vi "VP_RT_ModTrans.vi"() -> ()   [LabVIEW 2015]
uses:
  Local or Remote.ctl
  State Enum.ctl
  Command Enum.ctl
  Controller Type.ctl
  EPICS Command Control.ctl
  Plot options enum.ctl
  Stream SM states.ctl
  <vilib>/Platform/TimedLoop/XDataNode/timing_clust.ctl
  <vilib>/Platform/TimedLoop/XDataNode/nitl_modes.ctl
  <vilib>/Platform/TimedLoop/XDataNode/wakeup.ctl
  Data Write Control.ctl
  Data stream writer.vi
  <vilib>/Utility/error.llb/Error Cluster From Error Code.vi
  <vilib>/rvi/errors/niLvFpgaAdjustHostInterfaceError.vi
  <vilib>/rvi/interface/common/niFpgaWaitOnOcc.vi
  <vilib>/FPGAPlugInAG/Dynamic/niLvFpga_Reset_Dynamic.vi
  <vilib>/FPGAPlugInAG/Dynamic/niLvFpga_Abort_Dynamic.vi
  <vilib>/FPGAPlugInAG/Dynamic/niLvFpga_Close_Dynamic.vi
  Error stream writer.vi
  <vilib>/Platform/TimedLoop/XDataNode/XDataNode.xnode
  <vilib>/rvi/interface/nirviReadWriteControl/nirviReadWriteControl.xnode
  <vilib>/rvi/interface/nirviMethod/nirviMethod.xnode
  <vilib>/rvi/interface/nirviCloseFPGA/nirviCloseFPGA.xnode
  <vilib>/Platform/TimedLoop/XDataNode/XDNodeRunTimeDep.lvlib
  <vilib>/rvi/errors/niLvFpgaMergeErrorWithErrorCode.vi
  NiFpgaLv.dll
  <vilib>/rvi/interface/Simulation/niFpgaSimulationCallBeginRW.vi
  <vilib>/rvi/Analysis/host/Public/NI_FpgaMspHost.lvlib
  <vilib>/FPGAPlugInAG/Dynamic/niLvFpga_StopFifo_Dynamic.vi
  <vilib>/FPGAPlugInAG/Dynamic/niLvFpga_ReadFifo_Dynamic.vi
  <vilib>/NI_Real-Time Target Support.lvlib
  <vilib>/FPGAPlugInAG/Dynamic/niLvFpga_ConfigureFifo_Dynamic.vi
  <vilib>/FPGAPlugInAG/Dynamic/niLvFpga_StartFifo_Dynamic.vi
  <resource>/objmgr/ni.dex.rc
panel:
  in  "Tab Control":T1(tab)
  in  "Controller Type":T2
  in  "X Ramp Start (nm)":fxp<+/-,32,16>
  in  "X Ramp End (nm)":fxp<+/-,32,16>=500.0
  in  "Y Ramp Start (nm)":fxp<+/-,32,16>
  in  "Y Ramp End (nm)":fxp<+/-,32,16>=-500.0
  in  "Y Step Size (nm)":fxp<+/-,32,16>=50.0
  in  "X Step Size (nm)":fxp<+/-,32,16>=50.0
  in  "System Loop Type":enum16{"Open Loop", "Closed Loop"}(ring)=enum."Closed Loop"
  in  "DT Frequency (Hz)":dbl=3000.0 format="%#_6p"
  in  "DT duty cycle (%)":dbl=88.0 min=0.0 max=100.0 step=1.0
  in  "Max radius":fxp<+/-,32,16>=500.0
  in  "Spiral Step Size":fxp<+/-,32,16>=50.0
  in  "Scan Geometry":T3(ring)
  in  "Inner Scan axis":enum16{"X", "Y"}(ring)
  in  "Rotation Direction":enum16{"Clockwise", "Anti-clockwise"}(ring)
  in  "Radial direction":enum16{"Outward", "Inward"}(ring)
  out "Trajectory Completed":bool
  out "XY Ref":cluster{dbl[], dbl[]}[](graph)
  out "Elements Available in FIFO":u32(graph)
  out "Elements Remaining in FIFO":u32(graph)
  out "Reference and Actual positions":cluster{"t0":dbl, dbl, dbl[][]}(graph)
  in  "Timeout FPGA FIFO1":i32=40000000
  out "FIFO Timed Out":bool
  out "Stop Run":bool
  in  "Datalog Cases":T4(ring)=enum."Data Log 16"
  out "FIFO Timed Out?":bool
  out "Data Read Rate (Hz)":dbl=25000.000000000004
  out "Elements Remaining":u32
  in  "FIFO Timeout (ms)":i32=2500
  out "Actual Depth":u32=131068416
  in  "Requested Depth":u32=131068000
  in  "Fly scan loop dt":i64=250
  in  "Start Scan Loop dt":i64=50
  out "Queue is empty":bool=TRUE
  out "2iddVELO:VP:X_End_nm":dbl=2000.0
  out "2iddVELO:VP:X_Start_nm":dbl=-2000.0
  out "EPICS Execute Command":bool
  out "2iddVELO:VP:Y_Start_nm":dbl=2000.0
  out "2iddVELO:VP:Y_End_nm":dbl=-2000.0
  out "2iddVELO:VP:Y_Step_Size_nm":dbl=50.0
  out "2iddVELO:VP:X_Step_Size_nm":dbl=50.0
  out "2iddVELO:VP:Trigger_Freq_Hz":dbl=1000.0
  out "2iddVELO:VP:Trig_DutyCycle_Per":dbl=99.0
  out "Remote Mode":bool
  out "EPICS Controller Type":T2
  out "EPICS cRIO Command":T5
  out "EPICS Scan Trajectory":T3(ring)
  out "2iddVELO:VP:Max_Radius":dbl
  out "2iddVELO:VP:Spiral_Step":dbl
  out "Iteration Duration RT Timed-Loop":i64=128
  in  "Controller Time Period (uSec)":u32=40
  in  "Controller Output Time Period (uSec)":u32=40
  in  "XY Reference Time Period (uSec)":u32=40
  in  "Plant Output Time Period (uSec)":u32=40
  in  "Datalog Time Period (uSec)":u32=40
  in  "Trigger Generation Time Period (uSec)":u32=40
  in  "Z Reference Time Period (uSec)":u32=40
  in  "Stop System (Careful!!)":bool
  in  "Reset All":bool
  in  "Base name":string="base_name"
  out "Mod6/DIO3":bool
  out "Mod5/DIO3":bool
  out "Mod4/DIO3":bool
  in  "Sample Z Stage Resolution (nm)":fxp<+,33,3>=0.5
  in  "Sample Y Stage Resolution (nm)":fxp<+,33,3>=0.5
  in  "Sample X Stage Resolution (nm)":fxp<+,33,3>=0.5
  in  "Optics Z Stage Resolution (nm)":fxp<+,33,3>=0.5
  in  "Optics Y Stage Resolution (nm)":fxp<+,33,3>=0.5
  in  "Optics X Stage Resolution (nm)":fxp<+,33,3>=0.5
  in  "Sample Z Reset":bool
  in  "Sample Y Reset":bool
  in  "Sample X Reset":bool
  out "Mod6/DIO2":bool
  out "Mod6/DIO1":bool
  out "Mod6/DIO0":bool=TRUE
  out "Mod5/DIO2":bool
  out "Mod5/DIO1":bool=TRUE
  out "Mod5/DIO0":bool
  out "Mod4/DIO2":bool=TRUE
  out "Mod4/DIO1":bool
  out "Mod4/DIO0":bool=TRUE
  in  "Optics Z Reset":bool
  in  "Optics Y Reset":bool
  in  "Optics X Reset":bool
  out "Heartbeat":bool=TRUE
  in  "System command":T6
  in  "Execute":bool
  out "Last Command Executed":T6
  in  "Optics and or Sample Stage":T7(ring)
  in  "Local_Lock":bool
  out "Local or EPICS":T8
  out "Output filename":string
  out "Output path":path
  in  "cRIO data dir":string="/home/lvuser/natinst/data"
  out "RT Main Loop State":T9
  out "cRIO path":path
  out "Iteration Duration":i64
  out "EPICS rotation direction":enum16{"Clockwise", "Anti-clockwise"}(ring)
  out "EPICS radial direction":enum16{"Outward", "Inward"}(ring)
  out "EPICS Inner axis":enum16{"X", "Y"}(ring)
  out "Optics Z Stage Displacement (nm)":fxp<+/-,32,16>
  out "Optics Y Stage Displacement (nm)":fxp<+/-,32,16>
  out "Optics X Stage Displacement (nm)":fxp<+/-,32,16>=-1.0
  in  "Scan type":enum16{"Fly", "Step"}(ring)
  out "EPICS Scan Type":enum16{"Fly", "Step"}(ring)
  out "Scan Type and Geometry":T10(ring)
  out "Position Number":u32
  in  "Plot option":T11
  out "EPICS data save trigger":enum16{"Detector", "Trajectory"}(ring)
  out "Outer Loop iterations":i32
  out "Counter Loop iterations":i32
  out "Plant output loop iterations":i32
  out "Module output loop iterations":i32
  out "Trigger Generation Loop iterations":i32
  out "FIFO loop iterations":i32
  out "XY Reference Loop iterations":i32
  out "Z Reference Loop iterations":i32
  out "Controller loop iterations":i32
  out "FPGA state":T12(ring)
  out "EPICS system loop type":enum16{"Open Loop", "Closed Loop"}(ring)
  out "2iddVELO:LabView:ZPZ_Command":dbl
  out "2iddVELO:LabView:ZPY_Command":dbl
  out "2iddVELO:LabView:ZPX_Command":dbl
  out "Data sream sends":i32
  out "Error stream sends":i32
  out "Data stream writer connection":bool
  out "Error stream writer connection":bool
  out "Data stream state":T13
  out "Error stream state":T13
  in  "Data phase offset (deg)":dbl
  in  "Data frequency (Hz)":dbl=2500.0
  in  "Data duty cycle (%)":dbl=50.0
  in  "Data Trigger Reset":bool
  out "Data Frequency":fxp<+,32,0>
  out "Data Duty Cycle (periods)":fxp<+,32,0>
  out "Data Phase Offset (periods)":fxp<+,32,0>
  out "2iddVELO:VP:Data_Freq_Hz":dbl
  in  "Z-Stage Scaling Direction":fxp<+/-,3,3>=-1.0
  in  "Y-Stage Scaling Direction":fxp<+/-,3,3>=-1.0
  in  "Z-Stage nm to V Scaling":fxp<+/-,32,12>=0.0005397796630859375
  in  "Y-Stage nm to V Scaling":fxp<+/-,32,12>=0.0014200210571289062
  in  "X-Stage Scaling Direction":fxp<+/-,3,3>=-1.0
  in  "X-Stage nm to V Scaling":fxp<+/-,32,12>=0.0005359649658203125
  in  "Controller Output Lower Limit":fxp<+/-,20,5>=-5.0
  in  "Controller Output Upper Limit":fxp<+/-,20,5>=5.0
  in  "FPGA Wait Timer (ms)":u16=5
  in  "Pre-Scan pause (ms)":u32=2000
  in  "Readback Loop time between iterations (ms)":u32=10
  in  "Z Reference DC Offset (nm)":fxp<+/-,15,15>
  in  "Y Reference DC Offset (nm)":fxp<+/-,16,16>
  in  "X Reference DC Offset (nm)":fxp<+/-,16,16>
  in  "Z Reference Amplitude (nm)":fxp<+/-,40,17>
  in  "Y Reference Amplitude (nm)":fxp<+/-,40,17>=100.0
  in  "X Reference Amplitude (nm)":fxp<+/-,40,17>=100.0
  out "Trajectory frequency (periods/tick)":fxp<+,32,0>=1.25030055642128e-07 format="%#.5e"
  in  "Trajectory frequency (Hz)":dbl=25000.0 format="%#_6p"
  out "actual Traj frequency (Hz)":dbl format="%#_6p"
  in  "Data Save Flag":enum16{"Skip Data", "Save Data"}(ring)=enum."Save Data"
  in  "X Start Marker (nm)":fxp<+/-,32,16>
  in  "Y Start Marker (nm)":fxp<+/-,32,16>
  in  "Post-Scan pause (ms)":u32=2000
  in  "Detector Trigger Lower Limit (V)":fxp<+/-,20,5>
  in  "Detector Trigger Upper Limit (V)":fxp<+/-,20,5>=5.0
  out "Detector Trigger In Range?":bool=TRUE
  in  "Det Reference Amplitude (V)":fxp<+/-,40,17>=5.0
  in  "DT Reference DC Offset (V)":fxp<+/-,16,16>
  out "Det Frequency (periods/tick)":fxp<+,32,0>=7.500010542571545e-05
  out "Det Phase Offset (periods)":fxp<+,32,0>
  in  "Det Reset":bool
  out "Det Duty Cycle (periods)":fxp<+,32,0>=0.8799999998882413
  in  "Det phase offset (deg)":dbl format="%#.6g"
  out "Det Trigger Frequency (Hz)":dbl
  out "Det Trigger Duty Cycle (%)":dbl
  in  "Scaling mV to V":fxp<+,33,10>=0.001000046730041504
  out "Measured Datalog Time Period (Ticks)":u32=1600
  out "Measured Datalog Loop Rate (us)":dbl=3.9999999999999996e-05
  out "Measured Datalog Loop Rate (kHz)":dbl=25.000000000000004
  out "Measured Counter Loop Rate (us)":dbl
  out "Measured Counter Loop Rate (MHz)":dbl=inf
  out "Measured XY Reference Loop Rate (us)":dbl=3.9999999999999996e-05
  out "Measured XY Reference Loop Rate (kHz)":dbl=25.000000000000004
  out "Measured XY Reference Time Period (Ticks)":u32=1600
  out "Measured Controller Loop Rate (kHz)":dbl=25.000000000000004
  out "Measured Controller Output Loop Rate (us)":dbl=3.9999999999999996e-05
  out "Measured Controller Output Loop Rate (kHz)":dbl=25.000000000000004
  out "Measured Plant Output Loop Rate (us)":dbl=3.9999999999999996e-05
  out "Measured Plant Output Loop Rate (kHz)":dbl=25.000000000000004
  out "Measured Controller Loop Rate (us)":dbl=3.9999999999999996e-05
  out "Measured Controller Time Period (Ticks)":u32=1600
  out "Data Read Period (sec)":dbl=3.9999999999999996e-05
  out "Measured Controller Output Time Period (Ticks)":u32=1600
  out "Measured Plant Output Time Period (Ticks)":u32=1600
  out "Measured Counter Time Period (Ticks)":u32
  out "Measured Trigger Gen Time Period (Ticks)":u32=1600
  out "Measured Z Reference Time Period (Ticks)":u32=1600
  out "Measured Z Reference Loop Rate (us)":dbl=3.9999999999999996e-05
  out "Measured Z Reference Loop Rate (kHz)":dbl=25.000000000000004
  out "Number of Data Strings":i32=5
  out "Data":fxp<+/-,40,32>[](array[numeric])
  out "Measured Trigger Gen Loop Rate (us)":dbl=3.9999999999999996e-05
  out "Measured Trigger Gen Loop Rate (kHz)":dbl=25.000000000000004
  out "Z-Stage Input In Range?":bool=TRUE
  out "Y-Stage Input In Range?":bool=TRUE
  out "X-Stage Input In Range?":bool=TRUE
  out "Controller Output Upper Limit Readback":fxp<+/-,20,5>
  out "Kyy Output, Kyy*ey (V)":fxp<+/-,58,25>
  out "Controller Output Lower Limit Readback":fxp<+/-,20,5>
  out "Kxx Output, Kxx*ex (V)":fxp<+/-,58,25>
  out "Kzz Output, Kzz*ez (V)":fxp<+/-,58,25>
  in  "file path soscoeff_xx1 Hinf":path=path "/home/lvuser/natinst/controllers/Kxx_1_Gxx_matched_dow_16ord_mVpnm_cd8a3_AvTio9_X5nm_500pm_all_40us_soscof_xx1.mat"
  in  "file path sos gain SF Controller_xx1 Hinf":path=path "/home/lvuser/natinst/controllers/Kxx_1_Gxx_matched_dow_16ord_mVpnm_cd8a3_AvTio9_X5nm_500pm_all_40us_soscof_xx2.mat"
  in  "file path soscoeff_yy1 Hinf":path=path "/home/lvuser/natinst/controllers/Kyy_trial_1_Gyy_matched_dow_8ord_mVpnm_cd8a3_AvTio9_Y5nm_500pm_all_40us_soscof_yy1.mat"
  in  "file path sos gain SF Controller_yy1 Hinf":path=path "/home/lvuser/natinst/controllers/Kyy_trial_1_Gyy_matched_dow_8ord_mVpnm_cd8a3_AvTio9_Y5nm_500pm_all_40us_soscof_yy2.mat"
  in  "file path soscoeff_zz1 Hinf":path=path "/home/lvuser/natinst/controllers/Kzz_1_Gzz_matched_dow_29ord_mVpnm_cd8a3_AvTio9_Z5nm_500pm_all_40us_soscof_zz1.mat"
  in  "file path sos gain SF Controller_zz1 Hinf":path=path "/home/lvuser/natinst/controllers/Kzz_1_Gzz_matched_dow_29ord_mVpnm_cd8a3_AvTio9_Z5nm_500pm_all_40us_soscof_zz2.mat"
  in  "file path soscoeff_xx1 PID":path=path "/home/lvuser/natinst/controllers/Kxx_pid_2_Gxx_tustin_2ord_mVpnm_cd8a3_soscof_xx1.mat"
  in  "file path sos gain SF Controller_xx1 PID":path=path "/home/lvuser/natinst/controllers/Kxx_pid_2_Gxx_tustin_2ord_mVpnm_cd8a3_soscof_xx2.mat"
  in  "file path soscoeff_yy1 PID":path=path "/home/lvuser/natinst/controllers/Kyy_pid_4_Gyy_tustin_2ord_mVpnm_cd8a3_soscof_yy1.mat"
  in  "file path sos gain SF Controller_yy1 PID":path=path "/home/lvuser/natinst/controllers/Kyy_pid_4_Gyy_tustin_2ord_mVpnm_cd8a3_soscof_yy2.mat"
  in  "file path soscoeff_zz1 PID":path=path "/home/lvuser/natinst/controllers/Kzz_pid_2_Gzz_tustin_2ord_mVpnm_cd8a3_soscof_zz1.mat"
  in  "file path sos gain SF Controller_zz1 PID":path=path "/home/lvuser/natinst/controllers/Kzz_pid_2_Gzz_tustin_2ord_mVpnm_cd8a3_soscof_zz2.mat"
  out "-a01(2) xx1c":fxp<+/-,64,9>[](array[numeric])=[0.637785025840232, 0.9924182654286198, 1.8461027816316544, 0.8635404845716299, 1.0670555456779864, 1.6350703383821101, 1.6323955588345012, 1.1102241390539636, 0.0, 0.0, 0.0, 0.0, 0.0, 0.0, 0.0, 0.0, 0.0, 0.0, 0.0, 0.0]
  out "-a02(2) xx1c":fxp<+/-,64,9>[](array[numeric])=[-0.999855815746439, -0.9676991072632725, -0.9642268720534838, -0.9446498323360957, -0.9442808087139987, -0.7547983908829242, -0.6690016013017409, -0.11027986125857198, 0.0, 0.0, 0.0, 0.0, 0.0, 0.0, 0.0, 0.0, 0.0, 0.0, 0.0, 0.0]
  out "b01(2) xx1c":fxp<+/-,64,9>[](array[numeric])=[-0.6378105164532328, -1.0062332697665268, -1.8762916543815855, -0.8616288879491845, -1.0856571140792324, -1.6862585929720944, -1.743591709663851, -0.6129835805090948, 0.0, 0.0, 0.0, 0.0, 0.0, 0.0, 0.0, 0.0, 0.0, 0.0, 0.0, 0.0]
  out "b02(2) xx1c":fxp<+/-,64,9>[](array[numeric])=[0.9999102047610771, 0.9971375605901365, 0.9926840301018772, 0.9509648854364836, 0.9563369558920378, 0.7818900462139817, 0.7642575436257291, 3.0531133177191805e-16, 0.0, 0.0, 0.0, 0.0, 0.0, 0.0, 0.0, 0.0, 0.0, 0.0, 0.0, 0.0]
  out "sos gain SF Controller xx1c":fxp<+/-,42,9>=-0.1625035791657865
  out "-a01(2) yy1c":fxp<+/-,64,9>[](array[numeric])=[1.8740229377643998, 1.3096977339382483, 1.7453886241944765, 0.2668895009727739, 0.0, 0.0, 0.0, 0.0, 0.0, 0.0, 0.0, 0.0, 0.0, 0.0, 0.0, 0.0, 0.0, 0.0, 0.0, 0.0]
  out "-a02(2) yy1c":fxp<+/-,64,9>[](array[numeric])=[-0.9732703278433918, -0.5194903821190732, -0.7453924481836136, -2.7755575615628914e-17, 0.0, 0.0, 0.0, 0.0, 0.0, 0.0, 0.0, 0.0, 0.0, 0.0, 0.0, 0.0, 0.0, 0.0, 0.0, 0.0]
  out "b01(2) yy1c":fxp<+/-,64,9>[](array[numeric])=[-1.8979173162254057, -1.8463149313261074, -1.7151162246453355, -0.006444279582847878, 0.0, 0.0, 0.0, 0.0, 0.0, 0.0, 0.0, 0.0, 0.0, 0.0, 0.0, 0.0, 0.0, 0.0, 0.0, 0.0]
  out "b02(2) yy1c":fxp<+/-,64,9>[](array[numeric])=[0.9969084979865663, 0.9421233904433339, 0.7362048104846675, 0.0, 0.0, 0.0, 0.0, 0.0, 0.0, 0.0, 0.0, 0.0, 0.0, 0.0, 0.0, 0.0, 0.0, 0.0, 0.0, 0.0]
  out "sos gain SF Controller yy1c":fxp<+/-,42,9>=-1.480983349494636
  out "-a01(2) zz1c":fxp<+/-,64,9>[](array[numeric])=[0.6242394224317618, 1.8967038692417004, 0.6659160318030806, 1.7792660019034106, 1.6870099721477447, 0.6417945190222861, 1.4838029149808185, 1.8456549628851837, 1.2189509782386598, 0.9933314517253298, 1.0158915520299678, 0.8863484387433826, 0.026837806879254994, 1.8269783715122585, 0.22448441435364225, 0.0, 0.0, 0.0, 0.0, 0.0]
  out "-a02(2) zz1c":fxp<+/-,64,9>[](array[numeric])=[-0.9983298461163967, -0.9972287452752734, -0.995744457243837, -0.9947210838396919, -0.9925914602095722, -0.9920974045271405, -0.9881915357970101, -0.9800069383591395, -0.9760641145386646, -0.9508624135515895, -0.9242774595356998, -0.655945641403593, -0.008661844724279444, -0.8269827070369743, 0.0, 0.0, 0.0, 0.0, 0.0, 0.0]
  out "b01(2) zz1c":fxp<+/-,64,9>[](array[numeric])=[-0.6245671059510156, -1.897930093390194, -0.6670970070931089, -1.7670265604573054, -1.6833314913922348, -0.6327437892303018, -1.5025901530730128, -1.8636454269915796, -1.1210694827766767, -0.9982206064398196, -1.0326369335418408, -1.1342635673267367, -1.6852506306166828, -0.9843740162364313, -1.7208456881689926e-15, 0.0, 0.0, 0.0, 0.0, 0.0]
  out "b02(2) zz1c":fxp<+/-,64,9>[](array[numeric])=[0.9973135069419645, 0.9951302056171929, 0.9993435624612031, 0.9919371251860779, 0.994931751453586, 0.9881092761723503, 0.9884874399279107, 0.9977145546300196, 0.9725302934743221, 0.9855561672767964, 0.9893454712398023, 0.846212786518208, 0.7855598927779743, 0.0978075435519738, 0.0, 0.0, 0.0, 0.0, 0.0, 0.0]
  out "sos gain SF Controller zz1c":fxp<+/-,42,9>=-0.1988595259608701
  out "FPGA error monitor":errorcluster
  out "FPGA end run error":errorcluster
  out "Timed Loop (end error)":errorcluster
  out "Main Loop error":errorcluster
  out "Main Loop Iterations":i32
  out "RT error":errorcluster
  out "Command Loop Error":errorcluster
  out "Readback error":errorcluster
  out "FPGA wait error":errorcluster
  out "Coeff file import error":errorcluster
  out "Readback loop Iterations":i32
  out "Command Loop Iterations":i32
  out "Heartbeat Loop Iterations":i32
  out "EPICS command error":errorcluster
  out "FPGA Run Loop error":errorcluster
  out "File Writer loop error":errorcluster
  out "File writer loop iterations":i32
  out "Error stream writer iterations":i32
  out "Data stream writer iterations":i32
  out "Reduced Array of States":T9[](array[typedef])
  out "2iddVELO:VP:Scan_Type":string
  out "2iddVELO:VP:Controller_Type":string
  out "2iddVELO:VP:cRIO_Command":string
  out "2iddVELO:VP:Scan_Trajectory":string
  out "2iddVELO:VP:Radial_Direction":string
  out "2iddVELO:VP:Rotation_Direction":string
  out "2iddVELO:VP:Inner_Scan_Axis":string
  out "2iddVELO:VP:X_Center":dbl
  out "2iddVELO:VP:Y_Center":dbl
  out "2iddVELO:VP:Data_Save_Trigger":string
  out "2iddVELO:VP:System_Loop_Type":string
  out "Cleared Data":fxp<+/-,40,32>[](array[numeric])
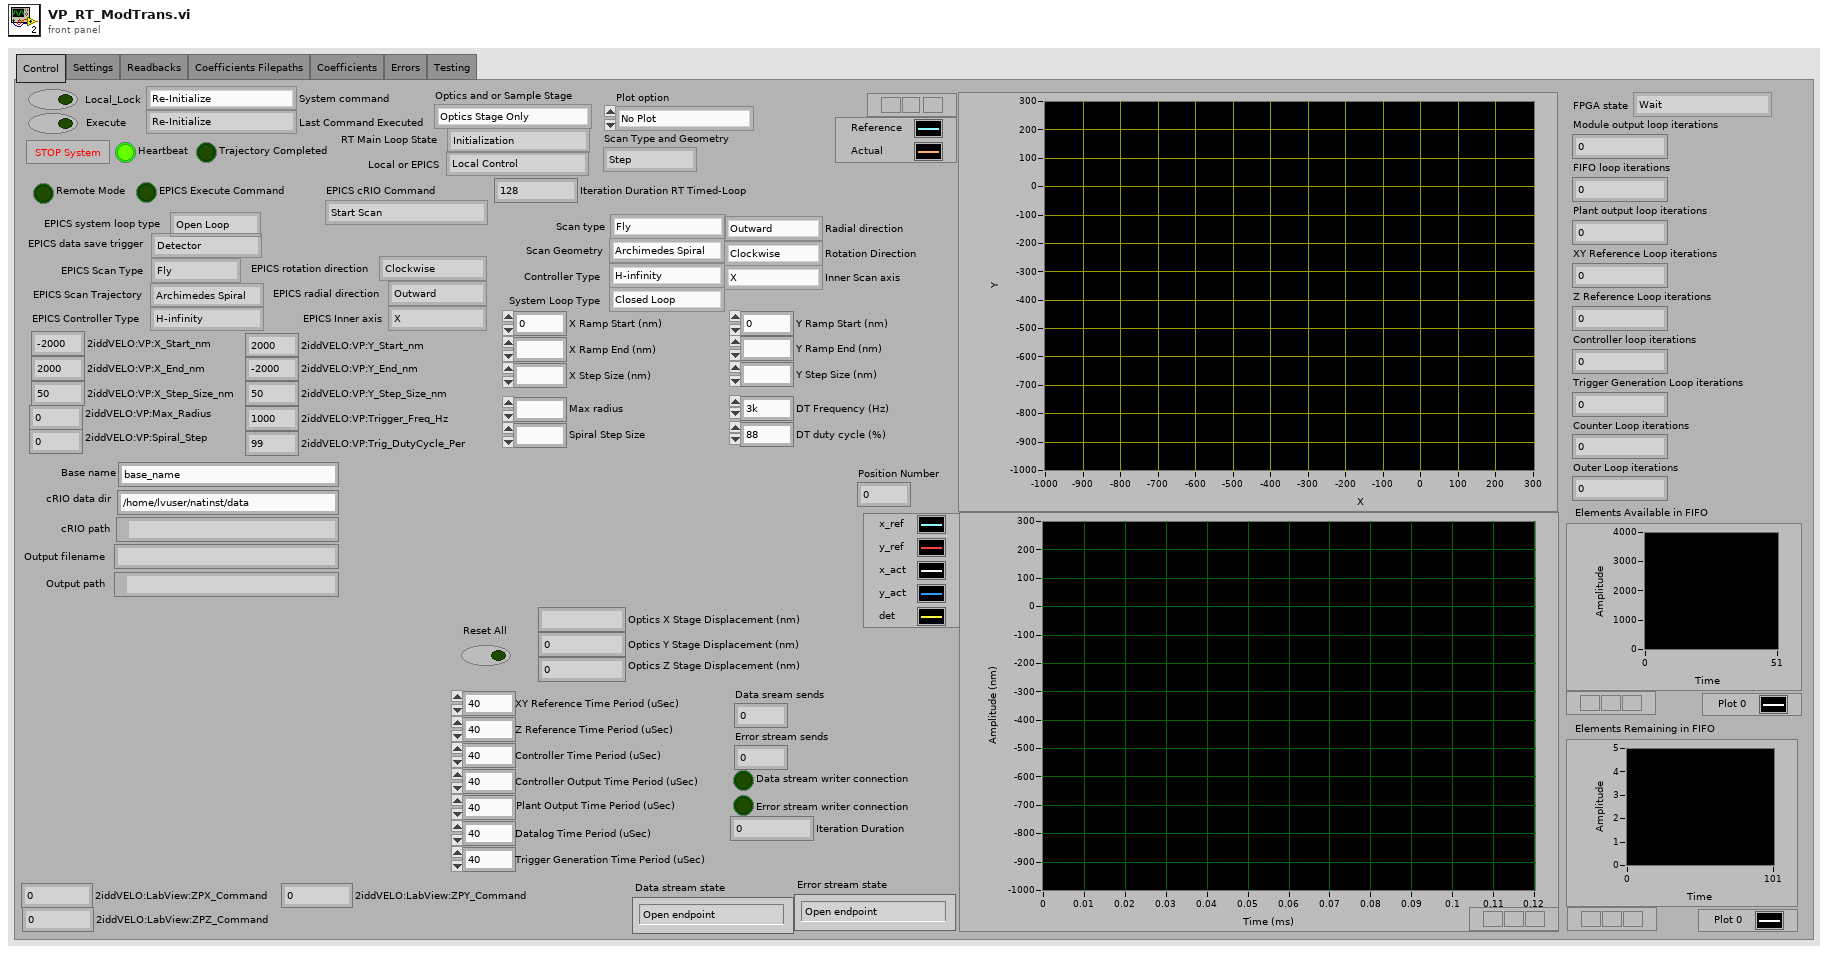
[diagram p1: front panel]
types:
  T1 = enum32{"Control", "Settings", "Readbacks", "Coefficients Filepaths", "Coefficients", "Errors", "Testing"}
  T2 = typedef "Controller Type.ctl" = enum16{"H-infinity", "PID"}
  T3 = enum16{"Archimedes Spiral", "Grid Spiral", "Snake"}
  T4 = enum16{"Data Log 1", "Data Log 2", "Data Log 3", "Data Log 4", "Data Log 5", "Data Log 6", "Data Log 7", "Data Log 8", "Data Log 9", "Data Log 10", "Data Log 11", "Data Log 12", "Data Log 13", "Data Log 14", "Data Log 15", "Data Log 16"}
  T5 = typedef "EPICS Command Control.ctl" = enum16{"Start Scan", "Stop Scan", "Reload Controller"}
  T6 = typedef "Command Enum.ctl" = enum16{"Re-Initialize ", "Update Scan Settings", "Scan", "Stop Scan", "Restart FPGA", "Stop System"}
  T7 = enum16{"Optics Stage Only", "Optics and Sample Stage"}
  T8 = typedef "Local or Remote.ctl" = enum16{"Local Control", "EPICS Control"}
  T9 = typedef "State Enum.ctl" = enum16{"Initialization", "Import Controller coeffs", "Update Controller Info", "Wait", "Update Reference Info", "Update Detector Trigger Info", "Update Datalog Info", "Check FPGA Status", "Initialize FIFO", "Pre-Scan", "Start Scan", "Step Scanning", "Fly Scanning", "End Scan", "Close File", "Restart FPGA", "Stop FPGA"}
  T10 = enum16{"Step", "Fly Arch Spiral", "Fly Snake", "Fly Grid Spiral"}
  T11 = typedef "Plot options enum.ctl" = enum16{"No Plot", "Partial Plot", "Full Plot"}
  T12 = enum16{"Wait", "Start Run", "Run", "End Run", "Shutdown"}
  T13 = typedef "Stream SM states.ctl" = enum16{"Open endpoint", "Wait", "ReadWrite", "Destroy endpoint"}
  T14 = typedef "XDNodeRunTimeDep.lvlib/timing_clust.ctl" = cluster{"Expected End [f-1]":u64, "Actual End [f-1]":u64, "Finished Late? [f-1]":bool, "Expected End [i-1]":u64, "Actual End [i-1]":u64, "Finished Late? [i-1]":bool, "Expected Start [i]":u64, "Actual Start [i]":u64, "Expected Start [f]":u64, "Actual Start [f]":u64, "Source Name":string, "Structure Name":string, "Period":i64, "Deadline":i64, "Offset":i64, "Start":i64, "Priority":i32, "Timeout":i32, "Mode":T15, "Wakeup Reason":T16, "Error":errorcluster, "Source Type":string, "Secondary Source Type":string, "Global End Time":u64, "Global Start Time":u64, "Frame Duration":u64, "Iteration Duration":u64, "Assigned CPU":i32, "I/O Scan Engine Mode":u32}
  T15 = typedef "XDNodeRunTimeDep.lvlib/nitl_modes.ctl" = enum32{"No Change", "Process missed periods, maintain original phase", "Discard missed periods, maintain original phase", "Process missed periods, ignore original phase", "Discard missed periods, ignore original phase"}
  T16 = typedef "XDNodeRunTimeDep.lvlib/wakeup.ctl" = enum32{"Normal", "Aborted", "Asynchronous wakeup", "Timing source error", "Timed loop error", "Timeout"}
  T17 = typedef "Data Write Control.ctl" = enum16{"Initialize", "Read", "Write", "Close"}
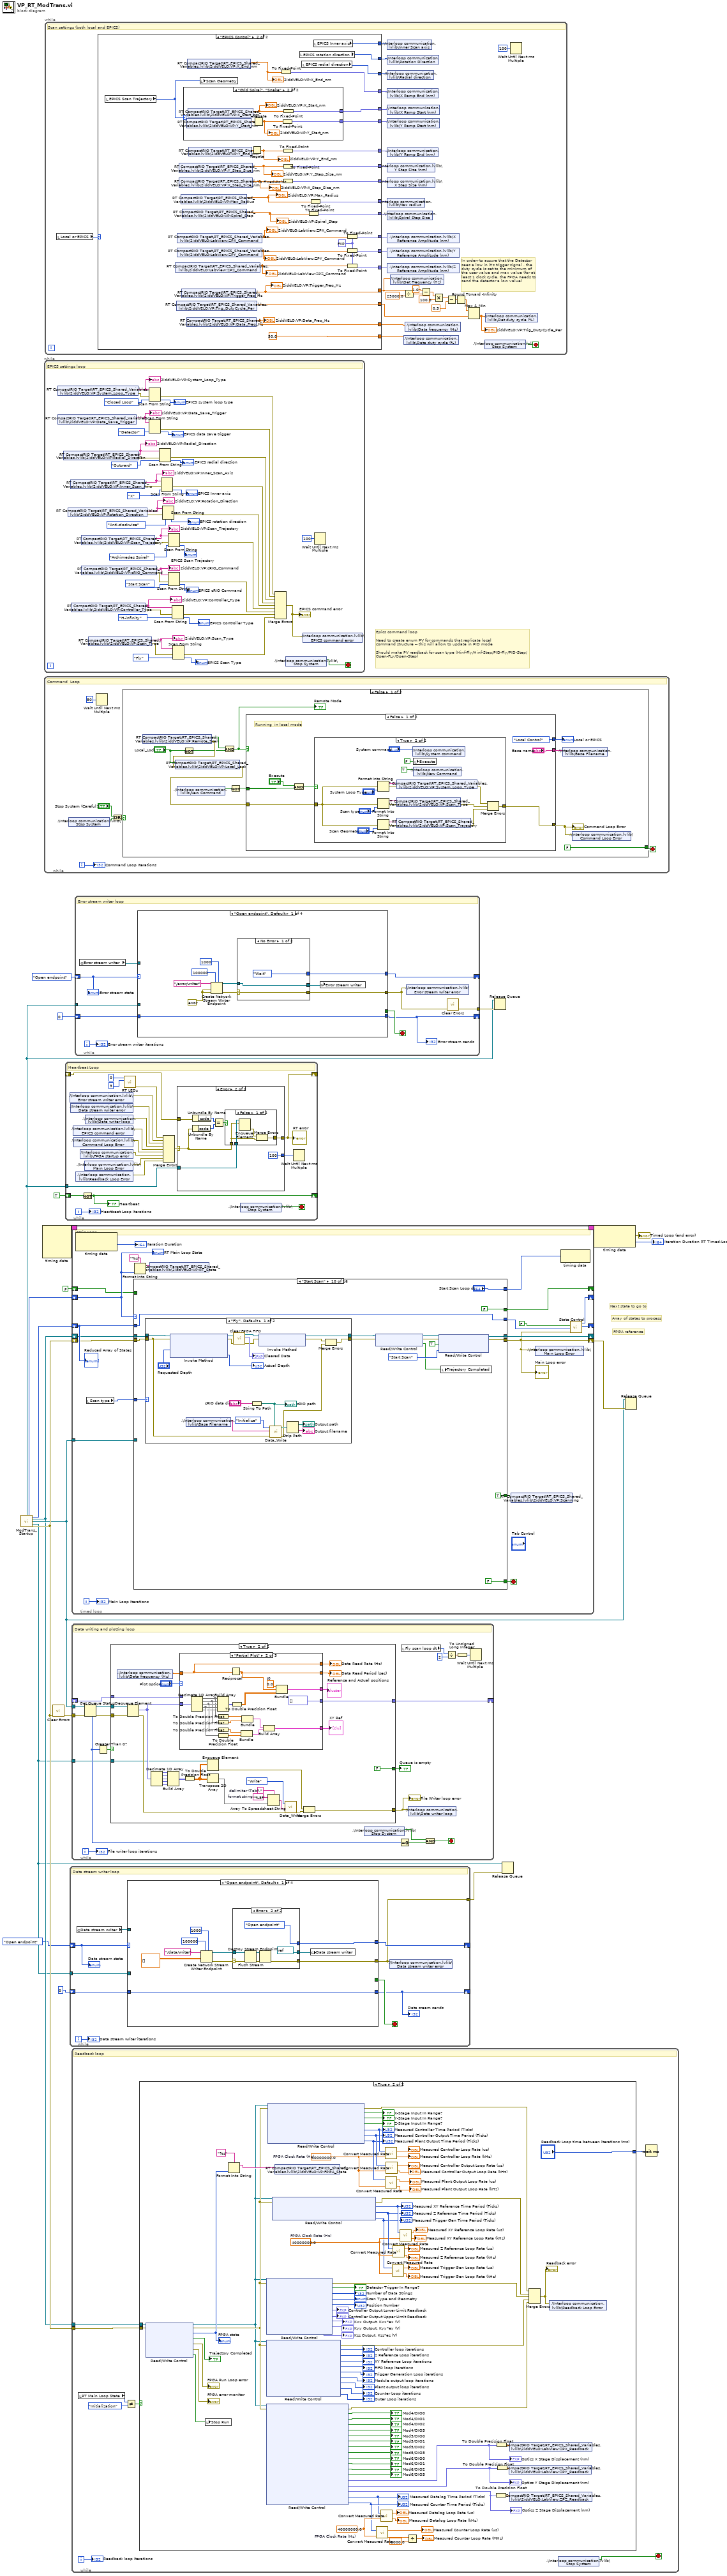
[diagram p0: block diagram]
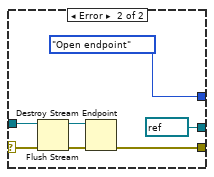
[diagram p2: hidden frame]
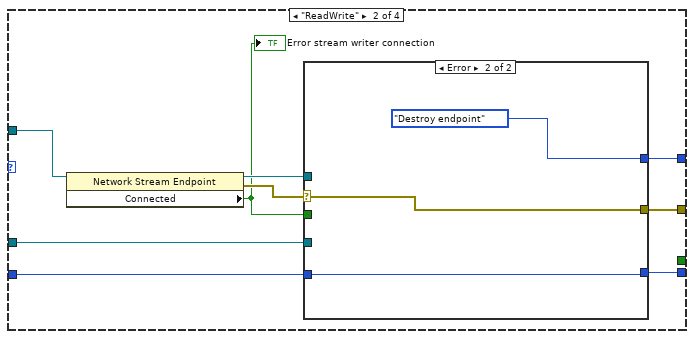
[diagram p3: hidden frame]
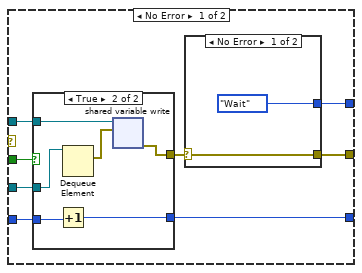
[diagram p4: hidden frame]
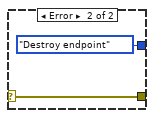
[diagram p5: hidden frame]
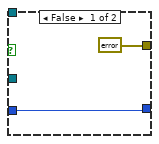
[diagram p6: hidden frame]
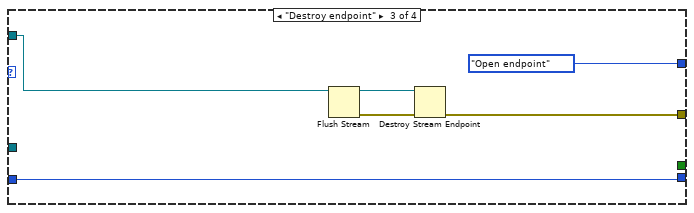
[diagram p7: hidden frame]
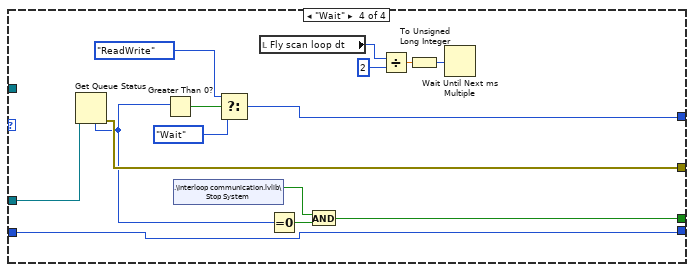
[diagram p8: hidden frame]
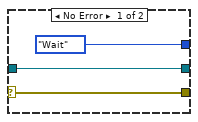
[diagram p9: hidden frame]
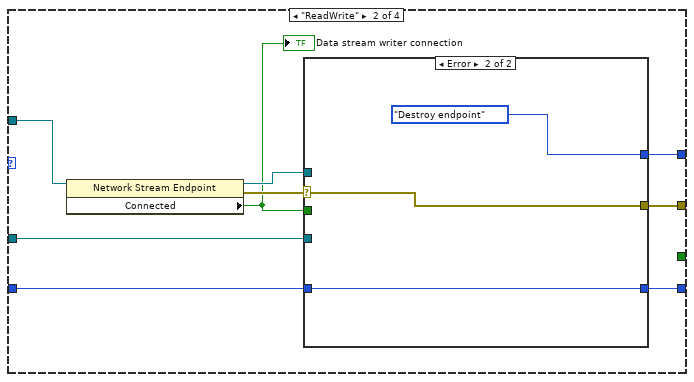
[diagram p10: hidden frame]
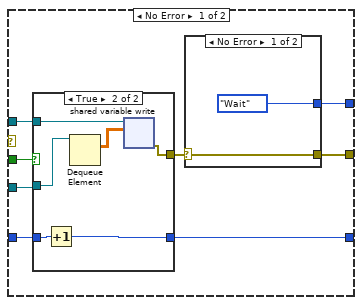
[diagram p11: hidden frame]
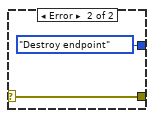
[diagram p12: hidden frame]
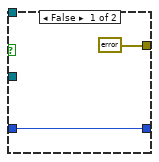
[diagram p13: hidden frame]
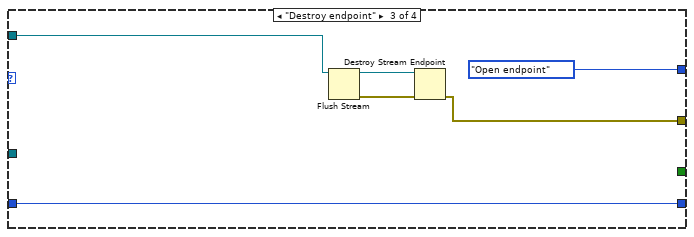
[diagram p14: hidden frame]
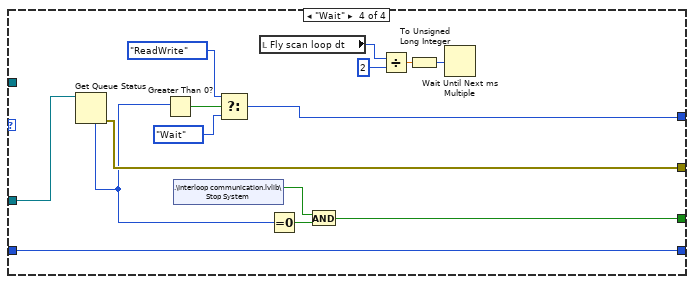
[diagram p15: hidden frame]
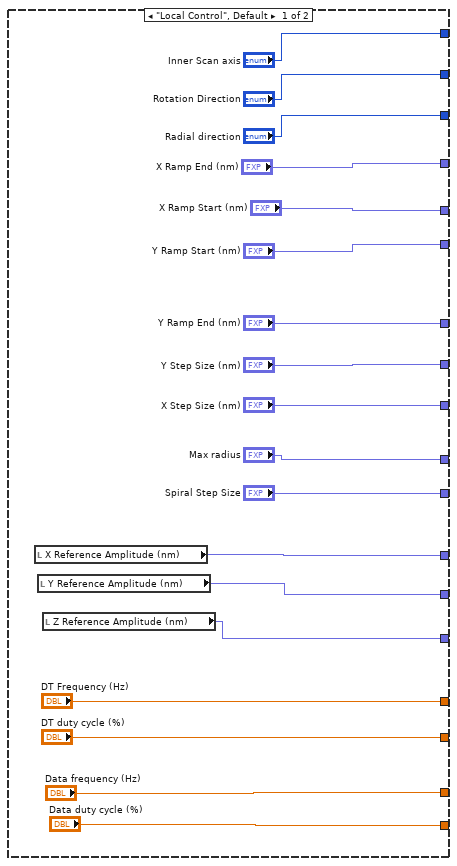
[diagram p16: hidden frame]
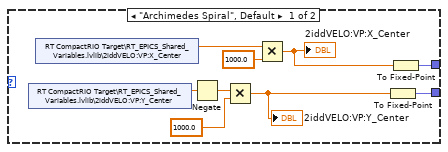
[diagram p17: hidden frame]
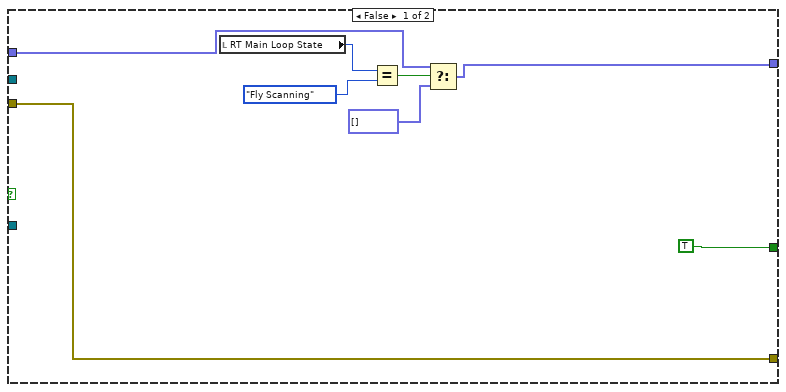
[diagram p18: hidden frame]
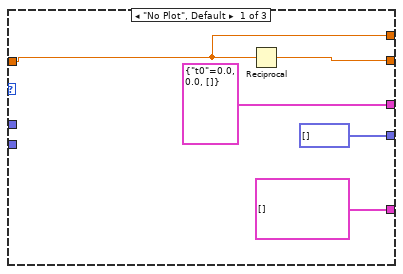
[diagram p19: hidden frame]
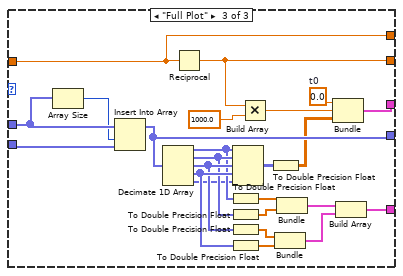
[diagram p20: hidden frame]
diagram:
  # "Epics command loop\n\nNeed to create enum PV for commands that replicate local\ncommand structure -- this will allow to update in PID mode\n\nShould make PV readback for scan type (Hinf-Fly/Hinf-Step/PID-Fly/PID-Step/\nOpen-FLy/Open-Step)"
  # "FPGA reference"
  # "Array of states to process"
  # "Next state to go to"
  n1 = call "ModTrans_Startup.vi"() -> ("Error stream queue"=w5:refnum<queue>, "States"=w12:T9, "Array of States"=w13:T9[], "Refnum out"=w10:refnum<k20>, "FIFO data queue"=w11:refnum<queue>, "Data stream queue"=w3:refnum<queue>, "error out"=w16:errorcluster)  [unwired: 9 in]
  n2 = node-c288() -> (w21:T14)  [unwired: 4 in]
  n3 = while {
    stop <- w22 stop-if-true
    # "EPICS settings loop"
    n4 = shared-variable "RT CompactRIO Target\\RT_EPICS_Shared_Variables.lvlib\\2iddVELO:VP:System_Loop_Type"() -> (w27:string, error out=w26:errorcluster)  [unwired: 1 in]
    "2iddVELO:VP:System_Loop_Type" <- w27
    n5 = shared-variable "RT CompactRIO Target\\RT_EPICS_Shared_Variables.lvlib\\2iddVELO:VP:Data_Save_Trigger"() -> (w31:string)  [unwired: 1 in, 1 out]
    "2iddVELO:VP:Data_Save_Trigger" <- w31
    n6 = shared-variable "RT CompactRIO Target\\RT_EPICS_Shared_Variables.lvlib\\2iddVELO:VP:Radial_Direction"() -> (w41:string, error out=w43:errorcluster)  [unwired: 1 in]
    "2iddVELO:VP:Radial_Direction" <- w41
    n7 = shared-variable "RT CompactRIO Target\\RT_EPICS_Shared_Variables.lvlib\\2iddVELO:VP:Rotation_Direction"() -> (w48:string, error out=w47:errorcluster)  [unwired: 1 in]
    "2iddVELO:VP:Rotation_Direction" <- w48
    n8 = shared-variable "RT CompactRIO Target\\RT_EPICS_Shared_Variables.lvlib\\2iddVELO:VP:Inner_Scan_Axis"() -> (w34:string, error out=w42:errorcluster)  [unwired: 1 in]
    "2iddVELO:VP:Inner_Scan_Axis" <- w34
    n9 = shared-variable "RT CompactRIO Target\\RT_EPICS_Shared_Variables.lvlib\\2iddVELO:VP:Controller_Type"() -> (w66:string, error out=w59:errorcluster)  [unwired: 1 in]
    "2iddVELO:VP:Controller_Type" <- w66
    n10 = shared-variable "RT CompactRIO Target\\RT_EPICS_Shared_Variables.lvlib\\2iddVELO:VP:Scan_Trajectory"() -> (w53:string, error out=w51:errorcluster)  [unwired: 1 in]
    "2iddVELO:VP:Scan_Trajectory" <- w53
    n11 = shared-variable "RT CompactRIO Target\\RT_EPICS_Shared_Variables.lvlib\\2iddVELO:VP:cRIO_Command"() -> (w65:string, error out=w61:errorcluster)  [unwired: 1 in]
    "2iddVELO:VP:cRIO_Command" <- w65
    n12 = shared-variable "RT CompactRIO Target\\RT_EPICS_Shared_Variables.lvlib\\2iddVELO:VP:Scan_Type"() -> (w64:string, error out=w57:errorcluster)  [unwired: 1 in]
    "2iddVELO:VP:Scan_Type" <- w64
    n13 = Scan From String(input string=w27, error in=w26, default 1=enum16{"Open Loop", "Closed Loop"}."Closed Loop" ("System Loop Type")) -> (error out=w25:errorcluster, output 1=→"EPICS system loop type":enum16{"Open Loop", "Closed Loop"})  [unwired: 2 in, 2 out]
    n14 = Scan From String(input string=w31, default 1=enum16{"Detector", "Trajectory"}."Detector" ("Data Save Trigger Source 2")) -> (error out=w30:errorcluster, output 1=→"EPICS data save trigger":enum16{"Detector", "Trajectory"})  [unwired: 3 in, 2 out]
    n15 = Scan From String(input string=w41, error in=w43, default 1=enum16{"Outward", "Inward"}."Outward" ("EPICS radial direction 2")) -> (error out=w44:errorcluster, output 1=→"EPICS radial direction":enum16{"Outward", "Inward"})  [unwired: 2 in, 2 out]
    n16 = Scan From String(input string=w34, error in=w42, default 1=enum16{"X", "Y"}."X" ("EPICS Inner axis 2")) -> (error out=w45:errorcluster, output 1=→"EPICS Inner axis":enum16{"X", "Y"})  [unwired: 2 in, 2 out]
    n17 = Scan From String(input string=w48, error in=w47, default 1=enum16{"Clockwise", "Anti-clockwise"}."Anti-clockwise" ("Rotation Direction 2")) -> (error out=w46:errorcluster, output 1=→"EPICS rotation direction":enum16{"Clockwise", "Anti-clockwise"})  [unwired: 2 in, 2 out]
    n18 = Scan From String(input string=w65, error in=w61, default 1=EPICS_Command_Control."Start Scan" ("default value 1")) -> (error out=w60:errorcluster, output 1=→"EPICS cRIO Command":T5)  [unwired: 2 in, 2 out]
    n19 = Scan From String(input string=w53, error in=w51, default 1=T3."Archimedes Spiral" ("Scan Geometry")) -> (error out=w50:errorcluster, output 1=→"EPICS Scan Trajectory":T3)  [unwired: 2 in, 2 out]
    n20 = Scan From String(input string=w66, error in=w59, default 1=Controller_Type."H-infinity" ("Controller Type")) -> (error out=w58:errorcluster, output 1=→"EPICS Controller Type":T2)  [unwired: 2 in, 2 out]
    n21 = Scan From String(input string=w64, error in=w57, default 1=enum16{"Fly", "Step"}."Fly" ("Scan type 2")) -> (error out=w56:errorcluster, output 1=→"EPICS Scan Type":enum16{"Fly", "Step"})  [unwired: 2 in, 2 out]
    n22 = Merge Errors(w25, w30, w44, w45, w46, w50, w60, w58, w56) -> (w55:errorcluster)
    "EPICS command error" <- w55
    n23 = shared-variable ".\\Interloop communication.lvlib\\Stop System"() -> (w22:bool)  [unwired: 1 in, 1 out]
    n24 = shared-variable ".\\Interloop communication.lvlib\\EPICS command error"(w55) -> ()  [unwired: 1 in, 1 out]
    n25 = Wait Until Next ms Multiple(millisecond multiple=u32 100) -> ()  [unwired: 1 out]
  }
  n26 = while {
    i -> [w72]
    stop <- w73 stop-if-true
    # "Command  Loop"
    n27 = shared-variable ".\\Interloop communication.lvlib\\Stop System"() -> (w71:bool)  [unwired: 1 in, 1 out]
    n28 = Wait Until Next ms Multiple(millisecond multiple=u32 50) -> ()  [unwired: 1 out]
    n29 = Or(x="Stop System (Careful!!)", y=w71) -> (x .or. y?=w70:bool)
    n30 = case shown="False" w70 {
      tunnel: [FALSE TRUE] -> w73
      frame False {
        n31 = shared-variable "RT CompactRIO Target\\RT_EPICS_Shared_Variables.lvlib\\2iddVELO:VP:Remote_Scan"() -> (w83:bool, error out=w81:errorcluster)  [unwired: 1 in]
        n32 = shared-variable "RT CompactRIO Target\\RT_EPICS_Shared_Variables.lvlib\\2iddVELO:VP:Local_Lock"("Local_Lock", error in=w81) -> (error out=w76:errorcluster)
        n33 = shared-variable ".\\Interloop communication.lvlib\\New Command"() -> (w86:bool)  [unwired: 1 in, 1 out]
        n34 = Not(x="Local_Lock") -> (.not. x?=w78:bool)
        n35 = And(x=w83, y=w78) -> (x .and. y?=w84:bool)
        "Remote Mode" <- w84
        n36 = Not(x=w86) -> (.not. x?=w85:bool)
        n37 = case shown="False" w84 {
          tunnel: w85 -> [w93 w120]
          tunnel: [Local_or_Remote."Local Control" ("Local or EPICS") Local_or_Remote."EPICS Control" ("Local or EPICS")] -> w75
          tunnel: w76 -> [w88 w115]
          tunnel: [w87 w118] -> w80
          tunnel: ["Base name" w117] -> w77
          frame False {
            # "Running  in local mode"
            n38 = And(x="Execute", y=w93) -> (x .and. y?=w91:bool)
            n39 = case shown="True" w91 {
              tunnel: w88 -> [w94 w101]
              tunnel: [w94 w95] -> w87
              frame False {
              }
              frame True {
                n40 = Format Into String(error in=w101, "System Loop Type") -> (resulting string=w103:string, error out=w104:errorcluster)  [unwired: 2 in]
                n41 = Format Into String(error in=w101, "Scan type") -> (resulting string=w100:string, error out=w107:errorcluster)  [unwired: 2 in]
                n42 = Format Into String(error in=w101, "Scan Geometry") -> (resulting string=w99:string, error out=w106:errorcluster)  [unwired: 2 in]
                n43 = shared-variable "RT CompactRIO Target\\RT_EPICS_Shared_Variables.lvlib\\2iddVELO:VP:System_Loop_Type"(w103, error in=w104) -> (error out=w98:errorcluster)
                n44 = shared-variable "RT CompactRIO Target\\RT_EPICS_Shared_Variables.lvlib\\2iddVELO:VP:Scan_Type"(w100, error in=w107) -> (error out=w97:errorcluster)
                n45 = shared-variable "RT CompactRIO Target\\RT_EPICS_Shared_Variables.lvlib\\2iddVELO:VP:Scan_Trajectory"(w99, error in=w106) -> (error out=w96:errorcluster)
                n46 = shared-variable ".\\Interloop communication.lvlib\\System command"("System command") -> ()  [unwired: 1 in, 1 out]
                n47 = local write "Execute"(FALSE ("Execute")) -> ()
                n48 = shared-variable ".\\Interloop communication.lvlib\\New Command"(TRUE ("New Command")) -> ()  [unwired: 1 in, 1 out]
                n49 = Merge Errors(w98, w97, w96) -> (w95:errorcluster)
              }
            }
          }
          frame True {
            # "Running in remote mode via EPICS PVs"
            n50 = shared-variable "RT CompactRIO Target\\RT_EPICS_Shared_Variables.lvlib\\2iddVELO:VP:Execute_Command"(error in=w115) -> (w116:bool, error out=w114:errorcluster)
            "EPICS Execute Command" <- w116
            n51 = shared-variable "RT CompactRIO Target\\RT_EPICS_Shared_Variables.lvlib\\2iddVELO:VP:Base_Filename"() -> (w117:string)  [unwired: 1 in, 1 out]
            n52 = And(x=w120, y=w116) -> (x .and. y?=w119:bool)
            n53 = case shown="True" w119 {
              tunnel: [w121 w129] -> w118
              tunnel: w114 -> [w121 w126]
              frame False {
              }
              frame True {
                n54 = local read "EPICS cRIO Command"() -> (w127:T5)
                n55 = shared-variable ".\\Interloop communication.lvlib\\New Command"(TRUE ("New Command")) -> ()  [unwired: 1 in, 1 out]
                n56 = shared-variable "RT CompactRIO Target\\RT_EPICS_Shared_Variables.lvlib\\2iddVELO:VP:Execute_Command"(FALSE ("2iddVELO:VP:Flyscan_Start"), error in=w126) -> (error out=w129:errorcluster)
                n57 = local read "EPICS Scan Type"() -> (w122:enum16{"Fly", "Step"})
                n58 = case shown="\"Stop Scan\"" w127 {
                  tunnel: [Command_Enum."Scan" ("System command") Command_Enum."Stop Scan" ("System command") Command_Enum."Re-Initialize " ("System command")] -> w124
                  frame "Start Scan", Default {
                  }
                  frame "Stop Scan" {
                  }
                  frame "Reload Controller" {
                  }
                }
                n59 = local read "EPICS system loop type"() -> (w123:enum16{"Open Loop", "Closed Loop"})
                n60 = local write "Scan type"(w122) -> ()
                n61 = shared-variable ".\\Interloop communication.lvlib\\System command"(w124) -> ()  [unwired: 1 in, 1 out]
                n62 = local write "System Loop Type"(w123) -> ()
              }
            }
            n63 = local write "Base name"(w117) -> ()
            n64 = local read "EPICS Controller Type"() -> (w113:T2)
            n65 = local write "Controller Type"(w113) -> ()
          }
        }
        "Local or EPICS" <- w75
        "Command Loop Error" <- w80
        n66 = shared-variable ".\\Interloop communication.lvlib\\Base Filename"(w77) -> ()  [unwired: 1 in, 1 out]
        n67 = shared-variable ".\\Interloop communication.lvlib\\Command Loop Error"(w80) -> ()  [unwired: 1 in, 1 out]
      }
      frame True {
        n68 = shared-variable ".\\Interloop communication.lvlib\\System command"(Command_Enum."Stop System" ("System command")) -> (error out=w133:errorcluster)  [unwired: 1 in]
        n69 = shared-variable ".\\Interloop communication.lvlib\\New Command"(TRUE ("New Command"), error in=w133) -> ()  [unwired: 1 out]
      }
    }
    "Command Loop Iterations" <- w72
  }
  n70 = while {
    stop <- w137 stop-if-true
    # "In orderr to assure that the Detector\nsees a low in it's trigger signal , the \nduty cycle is set to the minimum of \nthe user value and max value (for at\nleast 1 clock cycle, the FPGA needs to\nsend the detector a low value)"
    # "Scan settings (both local and EPICS)"
    n71 = local read "Local or EPICS"() -> (w167:T8)
    n72 = case shown="\"EPICS Control\"" w167 {
      tunnel: ["DT Frequency (Hz)" w215] -> w148
      tunnel: ["DT duty cycle (%)" w214] -> w150
      tunnel: [w181 w208] -> w166
      tunnel: [w182 w209] -> w165
      tunnel: [w183 w210] -> w164
      tunnel: ["Inner Scan axis" w189] -> w163
      tunnel: ["Rotation Direction" w190] -> w162
      tunnel: ["Radial direction" w191] -> w161
      tunnel: ["X Ramp Start (nm)" w192] -> w160
      tunnel: ["X Ramp End (nm)" w193] -> w159
      tunnel: ["Y Ramp Start (nm)" w194] -> w158
      tunnel: ["Y Ramp End (nm)" w195] -> w157
      tunnel: ["Y Step Size (nm)" w196] -> w156
      tunnel: ["X Step Size (nm)" w197] -> w155
      tunnel: ["Max radius" w198] -> w154
      tunnel: ["Spiral Step Size" w199] -> w153
      tunnel: ["Data frequency (Hz)" w188] -> w152
      tunnel: ["Data duty cycle (%)" 50.0 ("Data duty cycle (%)")] -> w151
      frame "Local Control", Default {
        n73 = local read "X Reference Amplitude (nm)"() -> (w183:fxp<+/-,40,17>)
        n74 = local read "Y Reference Amplitude (nm)"() -> (w182:fxp<+/-,40,17>)
        n75 = local read "Z Reference Amplitude (nm)"() -> (w181:fxp<+/-,40,17>)
      }
      frame "EPICS Control" {
        w207 = fxp<+/-,40,17> 0.0 ("Z Reference Amplitude (nm)")
        n76 = local read "EPICS Scan Trajectory"() -> (w186:T3)
        n77 = shared-variable "RT CompactRIO Target\\RT_EPICS_Shared_Variables.lvlib\\2iddVELO:LabView:ZPZ_Command"() -> (w213:dbl)  [unwired: 1 in, 1 out]
        "2iddVELO:LabView:ZPZ_Command" <- w213
        n78 = shared-variable "RT CompactRIO Target\\RT_EPICS_Shared_Variables.lvlib\\2iddVELO:VP:Trig_DutyCycle_Per"() -> (w214:dbl)  [unwired: 1 in, 1 out]
        n79 = shared-variable "RT CompactRIO Target\\RT_EPICS_Shared_Variables.lvlib\\2iddVELO:LabView:ZPY_Command"() -> (w212:dbl)  [unwired: 1 in, 1 out]
        "2iddVELO:LabView:ZPY_Command" <- w212
        n80 = shared-variable "RT CompactRIO Target\\RT_EPICS_Shared_Variables.lvlib\\2iddVELO:LabView:ZPX_Command"() -> (w211:dbl)  [unwired: 1 in, 1 out]
        "2iddVELO:LabView:ZPX_Command" <- w211
        n81 = shared-variable "RT CompactRIO Target\\RT_EPICS_Shared_Variables.lvlib\\2iddVELO:VP:Y_Step_Size_nm"() -> (w201:dbl)  [unwired: 1 in, 1 out]
        "2iddVELO:VP:Y_Step_Size_nm" <- w201
        n82 = shared-variable "RT CompactRIO Target\\RT_EPICS_Shared_Variables.lvlib\\2iddVELO:VP:X_Step_Size_nm"() -> (w202:dbl)  [unwired: 1 in, 1 out]
        "2iddVELO:VP:X_Step_Size_nm" <- w202
        n83 = shared-variable "RT CompactRIO Target\\RT_EPICS_Shared_Variables.lvlib\\2iddVELO:VP:Max_Radius"() -> (w206:dbl)  [unwired: 1 in, 1 out]
        "2iddVELO:VP:Max_Radius" <- w206
        n84 = shared-variable "RT CompactRIO Target\\RT_EPICS_Shared_Variables.lvlib\\2iddVELO:VP:Trigger_Freq_Hz"() -> (w215:dbl)  [unwired: 1 in, 1 out]
        "2iddVELO:VP:Trigger_Freq_Hz" <- w215
        n85 = shared-variable "RT CompactRIO Target\\RT_EPICS_Shared_Variables.lvlib\\2iddVELO:VP:Spiral_Step"() -> (w205:dbl)  [unwired: 1 in, 1 out]
        "2iddVELO:VP:Spiral_Step" <- w205
        n86 = case shown="\"Grid Spiral\", \"Snake\"" w186 {
          tunnel: [w224 w227] -> w192
          tunnel: [w223 w226] -> w194
          frame "Archimedes Spiral", Default {
            n87 = shared-variable "RT CompactRIO Target\\RT_EPICS_Shared_Variables.lvlib\\2iddVELO:VP:Y_Center"() -> (w217:dbl)  [unwired: 1 in, 1 out]
            n88 = shared-variable "RT CompactRIO Target\\RT_EPICS_Shared_Variables.lvlib\\2iddVELO:VP:X_Center"() -> (w222:dbl)  [unwired: 1 in, 1 out]
            n89 = Negate(x=w217) -> (-x=w219:dbl)
            n90 = Multiply(x=w219, y=1000.0) -> (x*y=w216:dbl)
            "2iddVELO:VP:Y_Center" <- w216
            n91 = Multiply(x=w222, y=1000.0) -> (x*y=w220:dbl)
            "2iddVELO:VP:X_Center" <- w220
            n92 = To Fixed-Point(number=w216) -> (fixed-point=w223:fxp<+/-,32,16>)  [unwired: 1 in]
            n93 = To Fixed-Point(number=w220) -> (fixed-point=w224:fxp<+/-,32,16>)  [unwired: 1 in]
          }
          frame "Grid Spiral", "Snake" {
            n94 = shared-variable "RT CompactRIO Target\\RT_EPICS_Shared_Variables.lvlib\\2iddVELO:VP:Y_Start_nm"() -> (w228:dbl)  [unwired: 1 in, 1 out]
            n95 = shared-variable "RT CompactRIO Target\\RT_EPICS_Shared_Variables.lvlib\\2iddVELO:VP:X_Start_nm"() -> (w229:dbl)  [unwired: 1 in, 1 out]
            "2iddVELO:VP:X_Start_nm" <- w229
            n96 = Negate(x=w228) -> (-x=w225:dbl)
            "2iddVELO:VP:Y_Start_nm" <- w225
            n97 = To Fixed-Point(number=w225) -> (fixed-point=w226:fxp<+/-,32,16>)  [unwired: 1 in]
            n98 = To Fixed-Point(number=w229) -> (fixed-point=w227:fxp<+/-,32,16>)  [unwired: 1 in]
          }
        }
        n99 = shared-variable "RT CompactRIO Target\\RT_EPICS_Shared_Variables.lvlib\\2iddVELO:VP:Data_Freq_Hz"() -> (w188:dbl)  [unwired: 1 in, 1 out]
        "2iddVELO:VP:Data_Freq_Hz" <- w188
        n100 = shared-variable "RT CompactRIO Target\\RT_EPICS_Shared_Variables.lvlib\\2iddVELO:VP:X_End_nm"() -> (w200:dbl)  [unwired: 1 in, 1 out]
        "2iddVELO:VP:X_End_nm" <- w200
        n101 = shared-variable "RT CompactRIO Target\\RT_EPICS_Shared_Variables.lvlib\\2iddVELO:VP:Y_End_nm"() -> (w203:dbl)  [unwired: 1 in, 1 out]
        n102 = local write "Scan Geometry"(w186) -> ()
        n103 = Negate(x=w203) -> (-x=w204:dbl)
        "2iddVELO:VP:Y_End_nm" <- w204
        n104 = To Fixed-Point(number=w200) -> (fixed-point=w193:fxp<+/-,32,16>)  [unwired: 1 in]
        n105 = To Fixed-Point(number=w204) -> (fixed-point=w195:fxp<+/-,32,16>)  [unwired: 1 in]
        n106 = To Fixed-Point(number=w201) -> (fixed-point=w196:fxp<+/-,32,16>)  [unwired: 1 in]
        n107 = To Fixed-Point(number=w202) -> (fixed-point=w197:fxp<+/-,32,16>)  [unwired: 1 in]
        n108 = local read "EPICS rotation direction"() -> (w190:enum16{"Clockwise", "Anti-clockwise"})
        n109 = local read "EPICS radial direction"() -> (w191:enum16{"Outward", "Inward"})
        n110 = To Fixed-Point(number=w205) -> (fixed-point=w199:fxp<+/-,32,16>)  [unwired: 1 in]
        n111 = To Fixed-Point(number=w206) -> (fixed-point=w198:fxp<+/-,32,16>)  [unwired: 1 in]
        n112 = local read "EPICS Inner axis"() -> (w189:enum16{"X", "Y"})
        n113 = To Fixed-Point(fixed-point type=w207, number=w211) -> (fixed-point=w210:fxp<+/-,40,17>)
        n114 = To Fixed-Point(fixed-point type=w207, number=w212) -> (fixed-point=w209:fxp<+/-,40,17>)
        n115 = To Fixed-Point(fixed-point type=w207, number=w213) -> (fixed-point=w208:fxp<+/-,40,17>)
      }
    }
    n116 = shared-variable ".\\Interloop communication.lvlib\\Inner Scan axis"(w163) -> ()  [unwired: 1 in, 1 out]
    n117 = shared-variable ".\\Interloop communication.lvlib\\Rotation Direction"(w162) -> ()  [unwired: 1 in, 1 out]
    n118 = shared-variable ".\\Interloop communication.lvlib\\Radial direction"(w161) -> ()  [unwired: 1 in, 1 out]
    n119 = shared-variable ".\\Interloop communication.lvlib\\X Ramp End (nm)"(w159) -> ()  [unwired: 1 in, 1 out]
    n120 = shared-variable ".\\Interloop communication.lvlib\\X Ramp Start (nm)"(w160) -> ()  [unwired: 1 in, 1 out]
    n121 = shared-variable ".\\Interloop communication.lvlib\\Y Ramp Start (nm)"(w158) -> ()  [unwired: 1 in, 1 out]
    n122 = shared-variable ".\\Interloop communication.lvlib\\Y Ramp End (nm)"(w157) -> ()  [unwired: 1 in, 1 out]
    n123 = shared-variable ".\\Interloop communication.lvlib\\Y Step Size (nm)"(w156) -> ()  [unwired: 1 in, 1 out]
    n124 = shared-variable ".\\Interloop communication.lvlib\\X Step Size (nm)"(w155) -> ()  [unwired: 1 in, 1 out]
    n125 = shared-variable ".\\Interloop communication.lvlib\\Max radius"(w154) -> ()  [unwired: 1 in, 1 out]
    n126 = shared-variable ".\\Interloop communication.lvlib\\Spiral Step Size"(w153) -> ()  [unwired: 1 in, 1 out]
    n127 = shared-variable ".\\Interloop communication.lvlib\\X Reference Amplitude (nm)"(w164) -> ()  [unwired: 1 in, 1 out]
    n128 = shared-variable ".\\Interloop communication.lvlib\\Y Reference Amplitude (nm)"(w165) -> ()  [unwired: 1 in, 1 out]
    n129 = shared-variable ".\\Interloop communication.lvlib\\Z Reference Amplitude (nm)"(w166) -> ()  [unwired: 1 in, 1 out]
    n130 = shared-variable ".\\Interloop communication.lvlib\\Det Frequency (Hz)"(w148) -> ()  [unwired: 1 in, 1 out]
    n131 = Divide(x=w148, y=25000.0) -> (x/y=w146:dbl)
    n132 = shared-variable ".\\Interloop communication.lvlib\\Data duty cycle (%)"(w151) -> ()  [unwired: 1 in, 1 out]
    n133 = shared-variable ".\\Interloop communication.lvlib\\Data frequency (Hz)"(w152) -> ()  [unwired: 1 in, 1 out]
    n134 = Subtract(x=1.0, y=w146) -> (x-y=w144:dbl)
    n135 = Multiply(x=w144, y=100.0) -> (x*y=w142:dbl)
    n136 = Subtract(x=w142, y=0.5) -> (x-y=w140:dbl)
    n137 = Round Toward -Infinity(1:w140) -> (0:w141:dbl)
    n138 = Max & Min(x=w141, y=w150) -> (min(x,y)=w149:dbl)  [unwired: 1 out]
    "2iddVELO:VP:Trig_DutyCycle_Per" <- w149
    n139 = shared-variable ".\\Interloop communication.lvlib\\Stop System"() -> (w137:bool)  [unwired: 1 in, 1 out]
    n140 = shared-variable ".\\Interloop communication.lvlib\\Det duty cycle (%)"(w149) -> ()  [unwired: 1 in, 1 out]
    n141 = Wait Until Next ms Multiple(millisecond multiple=u32 100) -> ()  [unwired: 1 out]
  }
  n142 = call <vilib>:"Clear Errors.vi"("error in (no error)"=w16) -> ("error out"=w9:errorcluster)  [unwired: 5 in, 1 out]
  n143 = while {
    shift-right: [w248] -> _
    shift-left: TRUE -> [w249]
    tunnel: w5 -> [w236]
    shift-right: [w231] -> _
    shift-left: _ -> [w230]
    i -> [w239]
    stop <- w237 stop-if-true
    # "Heartbeat Loop"
    n144 = shared-variable ".\\Interloop communication.lvlib\\Error stream writer error"() -> (w232:errorcluster)  [unwired: 1 in, 1 out]
    n145 = shared-variable ".\\Interloop communication.lvlib\\Data stream writer error"() -> (w233:errorcluster)  [unwired: 1 in, 1 out]
    n146 = shared-variable ".\\Interloop communication.lvlib\\EPICS command error"() -> (w238:errorcluster)  [unwired: 1 in, 1 out]
    n147 = shared-variable ".\\Interloop communication.lvlib\\Command Loop Error"() -> (w244:errorcluster)  [unwired: 1 in, 1 out]
    n148 = shared-variable ".\\Interloop communication.lvlib\\Readback Loop Error"() -> (w243:errorcluster)  [unwired: 1 in, 1 out]
    n149 = shared-variable ".\\Interloop communication.lvlib\\FPGA startup error"() -> (w242:errorcluster)  [unwired: 1 in, 1 out]
    n150 = Not(x=w249) -> (.not. x?=w248:bool)
    "Heartbeat" <- w248
    n151 = shared-variable ".\\Interloop communication.lvlib\\Main Loop Error"() -> (w247:errorcluster)  [unwired: 1 in, 1 out]
    n152 = shared-variable ".\\Interloop communication.lvlib\\Data writer loop"() -> (w235:errorcluster)  [unwired: 1 in, 1 out]
    n153 = call <vilib>:"RT LEDs.vi"("State"=3, "LED Num"=0) -> ("error out"=w234:errorcluster)  [unwired: 4 in, 1 out]
    n154 = Merge Errors(w234, w232, w233, w235, w238, w244, w242, w247, w243) -> (w245:errorcluster)
    n155 = case shown="Error" w245 {
      selector: w245 -> [w250 w254]
      tunnel: [u32 500 ("millisecond multiple") u32 100 ("millisecond multiple")] -> w246
      tunnel: [w250 w252] -> w231
      tunnel: w236 -> [_ w258]
      tunnel: w230 -> [_ w257]
      frame No Error {
      }
      frame Error {
        n156 = Unbundle By Name(w254) -> ("code"=w255:i32)
        n157 = Unbundle By Name(w257) -> ("code"=w256:i32)
        n158 = Equal?(x=w256, y=w255) -> (x = y?=w253:bool)
        n159 = case shown="False" w253 {
          tunnel: w258 -> [w263 _]
          tunnel: w254 -> [w260 w264]
          tunnel: [w262 w264] -> w252
          frame False {
            n160 = Enqueue Element(queue=w263, element=w260) -> (error out=w261:errorcluster)  [unwired: 2 in, 2 out]
            n161 = Merge Errors(w261, w260) -> (w262:errorcluster)
          }
          frame True {
          }
        }
      }
    }
    "RT error" <- w231
    n162 = shared-variable ".\\Interloop communication.lvlib\\Stop System"() -> (w237:bool)  [unwired: 1 in, 1 out]
    n163 = Wait Until Next ms Multiple(millisecond multiple=w246) -> ()  [unwired: 1 out]
    "Heartbeat Loop Iterations" <- w239
  }
  n164 = while {
    tunnel: w3 -> [w273]
    shift-right: [w272] -> _
    shift-left: Stream_SM_states."Open endpoint" -> [w265]
    tunnel: [w268] -> w4
    shift-right: [w266] -> _
    shift-left: 0 -> [w267]
    i -> [w270]
    stop <- w271 stop-if-true
    # "Data stream writer loop"
    n165 = global read "Data stream writer.vi" "Data stream writer"() -> (w269:refnum<k21>)
    n166 = case shown="\"Open endpoint\", Default" w265 {
      tunnel: w273 -> [_ w296 _ w346]
      tunnel: [w278 w299 Stream_SM_states."Open endpoint" ("f") w344] -> w272
      tunnel: [_ _ _ w335] -> w271
      tunnel: [w276 w298 w328 w334] -> w268
      tunnel: w269 -> [_ w297 w327 _]
      tunnel: w267 -> [w274 w295 w326 w333]
      tunnel: [w274 w294 w326 w333] -> w266
      frame "Open endpoint", Default {
        n167 = Create Network Stream Writer Endpoint(5:1000 ("timeout in ms (-1)"), 7:100000 ("writer buffer size"), 9:dbl[][] [], 11:"/data/writer" ("reader url")) -> (0:w279:errorcluster, 3:w277:refnum<k21>)  [unwired: 3 in]
        n168 = case shown="Error" w279 {
          selector: w279 -> [w285 w288]
          tunnel: [Stream_SM_states."Wait" Stream_SM_states."Open endpoint"] -> w278
          tunnel: w277 -> [w284 w290]
          tunnel: [w285 w287] -> w276
          tunnel: [w284 refnum<k21> refnum ("reader url")] -> w275
          frame No Error {
          }
          frame Error {
            n169 = Flush Stream(8:w288, 11:w290) -> (0:w291:errorcluster, 3:w289:refnum<k21>)  [unwired: 2 in, 1 out]
            n170 = Destroy Stream Endpoint(8:w291, 11:w289) -> (0:w287:errorcluster)
          }
        }
        n171 = global write "Data stream writer.vi" "Data stream writer"(w275) -> ()
      }
      frame "ReadWrite" {
        n172 = property class="Network Stream Endpoint"(reference=w297) -> (reference out=w302:refnum<k21>, error out=w301:errorcluster, "Connected"=w300:bool)  [unwired: 1 in]
        "Data stream writer connection" <- w300
        n173 = case shown="Error" w301 {
          selector: w301 -> [_ w325]
          tunnel: [w306 w325] -> w298
          tunnel: w302 -> [w310 _]
          tunnel: w300 -> [w309 _]
          tunnel: [w307 Stream_SM_states."Destroy endpoint"] -> w299
          tunnel: w296 -> [w305 _]
          tunnel: w295 -> [w304 w323]
          tunnel: [w303 w323] -> w294
          frame No Error {
            n174 = case shown="True" w309 {
              tunnel: [errorcluster {"status"=FALSE, "code"=0, "source"=""} ("error IO") w322] -> w308
              tunnel: w310 -> [_ w321]
              tunnel: w305 -> [_ w319]
              tunnel: w304 -> [w315 w318]
              tunnel: [w315 w317] -> w303
              frame False {
              }
              frame True {
                n175 = Increment(x=w318) -> (x+1=w317:i32)
                n176 = Dequeue Element(queue=w319) -> (element=w320:dbl[][])  [unwired: 2 in, 3 out]
                n177 = shared-variable-write(w321, w320) -> (w322:errorcluster)  [unwired: 2 in, 2 out]
              }
            }
            n178 = case shown="No Error" w308 {
              selector: w308 -> [w311 w313]
              tunnel: [Stream_SM_states."Wait" Stream_SM_states."Destroy endpoint"] -> w307
              tunnel: [w311 w313] -> w306
              frame No Error {
              }
              frame Error {
              }
            }
          }
          frame Error {
          }
        }
      }
      frame "Destroy endpoint" {
        n179 = Flush Stream(11:w327) -> (0:w330:errorcluster, 3:w331:refnum<k21>)  [unwired: 3 in, 1 out]
        n180 = Destroy Stream Endpoint(8:w330, 11:w331) -> (0:w328:errorcluster)
      }
      frame "Wait" {
        n181 = Get Queue Status(queue=w346) -> (error out=w334:errorcluster, # elements in queue=w332:i32)  [unwired: 2 in, 6 out]
        n182 = Greater Than 0?(x=w332) -> (x > 0?=w345:bool)
        n183 = shared-variable ".\\Interloop communication.lvlib\\Stop System"() -> (w337:bool)  [unwired: 1 in, 1 out]
        n184 = Select(t=Stream_SM_states."ReadWrite", s=w345, f=Stream_SM_states."Wait") -> (s? t:f=w344:T13)
        n185 = local read "Fly scan loop dt"() -> (w340:i64)
        n186 = Equal To 0?(x=w332) -> (x = 0?=w336:bool)
        n187 = And(x=w337, y=w336) -> (x .and. y?=w335:bool)
        n188 = Divide(x=w340, y=i64 2) -> (x/y=w339:dbl)
        n189 = To Unsigned Long Integer(number=w339) -> (unsigned 32bit integer=w341:u32)
        n190 = Wait Until Next ms Multiple(millisecond multiple=w341) -> ()  [unwired: 1 out]
      }
    }
    "Data sream sends" <- w266
    n191 = shared-variable ".\\Interloop communication.lvlib\\Data stream writer error"(w268) -> ()  [unwired: 1 in, 1 out]
    "Data stream writer iterations" <- w270
    "Data stream state" <- w265
  }
  n192 = timed-loop {
    timing: w21 -> [_]
    timing-out: [_] -> w20
    shift-right: [w348] -> _
    shift-left: w12 -> [w354]
    shift-right: [w365] -> _
    shift-left: w10 -> [w359]
    shift-right: [w358] -> w15
    shift-left: w16 -> [w360]
    shift-right: [w362] -> _
    shift-left: w13 -> [w363]
    tunnel: w11 -> [w352]
    shift-right: [w349] -> _
    shift-left: FALSE -> [w350]
    i -> [w364]
    stop <- w367 stop-if-true
    # "Main Loop"
    n193 = node-c288() -> (→"Iteration Duration":i64)  [unwired: 1 in, 1 out]
    n194 = local read "Scan type"() -> (w353:enum16{"Fly", "Step"})
    n195 = case shown="\"Start Scan\"" w354 {
      tunnel: [w376 w390 w433 w489 w547 w576 w597 w610 w636 w668 w718 w732 w765 w807 w837 w852] -> w366
      tunnel: [FALSE ("Stop") FALSE ("Stop") FALSE ("Stop") FALSE ("Stop") FALSE ("Stop") FALSE ("Stop") FALSE ("Stop") FALSE ("Stop") _ FALSE ("Stop") FALSE ("Stop") FALSE ("Stop") FALSE ("Stop") FALSE ("Stop") FALSE ("Stop") TRUE ("Stop")] -> w367
      tunnel: [w377 w395 w432 w491 w546 w575 w596 w612 w624 w677 w711 w726 w757 w803 w832 w849] -> w365
      tunnel: [w373 w392 w431 w485 w545 w574 w595 w603 w623 w676 w710 w746 w756 w798 w831 w854] -> w358
      tunnel: w360 -> [w370 w387 w435 w486 w540 w570 w598 w613 w634 w680 w712 w729 w768 w804 w835 w858]
      tunnel: w359 -> [w371 w395 w434 w491 w548 w577 w599 w614 w635 w666 w713 w748 w770 w803 w841 w859]
      tunnel: w363 -> [w376 w390 w433 _ w547 w576 w597 w610 w636 w668 w719 w733 w765 w806 w837 _]
      tunnel: [i64 0 i64 0 i64 0 i64 50 i64 0 i64 0 i64 0 i64 0 i64 0 "Start Scan Loop dt" i64 50 "Fly scan loop dt" i64 0 i64 0 i64 0 i64 0] -> w361
      tunnel: w353 -> [_ _ _ w483 w538 _ _ _ w625 w679 _ _ w766 _ _ _]
      tunnel: w352 -> [_ _ _ _ _ _ _ _ _ _ _ w727 _ _ _ _]
      tunnel: w350 -> [_ _ _ _ _ _ _ _ _ _ _ w722 _ _ _ _]
      tunnel: [FALSE FALSE FALSE FALSE FALSE FALSE FALSE FALSE FALSE FALSE FALSE TRUE FALSE FALSE FALSE FALSE] -> w349
      tunnel: [FALSE ("2iddVELO:VP:Scanning") FALSE ("2iddVELO:VP:Scanning") FALSE ("2iddVELO:VP:Scanning") FALSE ("2iddVELO:VP:Scanning") FALSE ("2iddVELO:VP:Scanning") FALSE ("2iddVELO:VP:Scanning") FALSE ("2iddVELO:VP:Scanning") FALSE ("2iddVELO:VP:Scanning") TRUE ("2iddVELO:VP:Scanning") TRUE ("2iddVELO:VP:Scanning") TRUE ("2iddVELO:VP:Scanning") TRUE ("2iddVELO:VP:Scanning") TRUE ("2iddVELO:VP:Scanning") w799 FALSE ("2iddVELO:VP:Scanning") FALSE ("2iddVELO:VP:Scanning")] -> w347
      frame "Initialization", Default {
        n196 = xnode "Read/Write Control"("FPGA VI Reference In"=w371, "error in"=w370) -> ("FPGA VI Reference Out"=w377:refnum<k20>, "error out"=w373:errorcluster, "Wait error"=w372:errorcluster)
        "FPGA wait error" <- w372
        n197 = shared-variable ".\\Interloop communication.lvlib\\FPGA startup error"(w372) -> ()  [unwired: 1 in, 1 out]
      }
      frame "Import Controller coeffs" {
        n198 = case shown="\"H-infinity\", Default" "Controller Type" {
          tunnel: ["file path soscoeff_xx1 Hinf" "file path soscoeff_xx1 PID"] -> w386
          tunnel: ["file path sos gain SF Controller_xx1 Hinf" "file path sos gain SF Controller_xx1 PID"] -> w385
          tunnel: ["file path soscoeff_yy1 Hinf" "file path soscoeff_yy1 PID"] -> w384
          tunnel: ["file path sos gain SF Controller_yy1 Hinf" "file path sos gain SF Controller_yy1 PID"] -> w383
          tunnel: ["file path sos gain SF Controller_zz1 Hinf" "file path sos gain SF Controller_zz1 PID"] -> w382
          tunnel: ["file path soscoeff_zz1 Hinf" "file path soscoeff_zz1 PID"] -> w381
          frame "H-infinity", Default {
          }
          frame "PID" {
          }
        }
        n199 = call "Read_coeff.vi"("error in (no error)"=w387, "sos gain SF controller file path"=w385, "sos coeff file path"=w386) -> ("b02(2)"=→"b02(2) xx1c":fxp<+/-,64,9>[], "b01(2)"=→"b01(2) xx1c":fxp<+/-,64,9>[], "-a02(2)"=→"-a02(2) xx1c":fxp<+/-,64,9>[], "-a01(2)"=→"-a01(2) xx1c":fxp<+/-,64,9>[], "error out"=w388:errorcluster, "sos gain SF Controller"=→"sos gain SF Controller xx1c":fxp<+/-,42,9>)  [unwired: 3 in]
        n200 = call "Read_coeff.vi"("error in (no error)"=w387, "sos gain SF controller file path"=w383, "sos coeff file path"=w384) -> ("b02(2)"=→"b02(2) yy1c":fxp<+/-,64,9>[], "b01(2)"=→"b01(2) yy1c":fxp<+/-,64,9>[], "-a02(2)"=→"-a02(2) yy1c":fxp<+/-,64,9>[], "-a01(2)"=→"-a01(2) yy1c":fxp<+/-,64,9>[], "error out"=w389:errorcluster, "sos gain SF Controller"=→"sos gain SF Controller yy1c":fxp<+/-,42,9>)  [unwired: 3 in]
        n201 = call "Read_coeff.vi"("error in (no error)"=w387, "sos gain SF controller file path"=w382, "sos coeff file path"=w381) -> ("b02(2)"=→"b02(2) zz1c":fxp<+/-,64,9>[], "b01(2)"=→"b01(2) zz1c":fxp<+/-,64,9>[], "-a02(2)"=→"-a02(2) zz1c":fxp<+/-,64,9>[], "-a01(2)"=→"-a01(2) zz1c":fxp<+/-,64,9>[], "error out"=w391:errorcluster, "sos gain SF Controller"=→"sos gain SF Controller zz1c":fxp<+/-,42,9>)  [unwired: 3 in]
        n202 = Merge Errors(w388, w389, w391) -> (w392:errorcluster)
        "Coeff file import error" <- w392
      }
      frame "Update Controller Info" {
        n203 = local read "sos gain SF Controller yy1c"() -> (w463:fxp<+/-,42,9>)
        n204 = local read "sos gain SF Controller xx1c"() -> (w468:fxp<+/-,42,9>)
        n205 = local read "sos gain SF Controller zz1c"() -> (w461:fxp<+/-,42,9>)
        n206 = local read "-a01(2) yy1c"() -> (w467:fxp<+/-,64,9>[])
        n207 = local read "-a02(2) yy1c"() -> (w466:fxp<+/-,64,9>[])
        n208 = local read "-a01(2) xx1c"() -> (w472:fxp<+/-,64,9>[])
        n209 = local read "-a02(2) xx1c"() -> (w471:fxp<+/-,64,9>[])
        n210 = local read "-a01(2) zz1c"() -> (w462:fxp<+/-,64,9>[])
        n211 = local read "-a02(2) zz1c"() -> (w458:fxp<+/-,64,9>[])
        n212 = local read "b01(2) yy1c"() -> (w465:fxp<+/-,64,9>[])
        n213 = local read "b02(2) yy1c"() -> (w464:fxp<+/-,64,9>[])
        n214 = local read "b01(2) xx1c"() -> (w470:fxp<+/-,64,9>[])
        n215 = local read "b02(2) xx1c"() -> (w469:fxp<+/-,64,9>[])
        n216 = local read "b01(2) zz1c"() -> (w459:fxp<+/-,64,9>[])
        n217 = local read "b02(2) zz1c"() -> (w460:fxp<+/-,64,9>[])
        n218 = Or(x="Optics Z Reset", y="Reset All") -> (x .or. y?=w452:bool)
        n219 = Or(x="Sample Z Reset", y="Reset All") -> (x .or. y?=w449:bool)
        n220 = Or(x="Optics X Reset", y="Reset All") -> (x .or. y?=w456:bool)
        n221 = Or(x="Optics Y Reset", y="Reset All") -> (x .or. y?=w454:bool)
        n222 = Or(x="Sample X Reset", y="Reset All") -> (x .or. y?=w451:bool)
        n223 = Or(x="Sample Y Reset", y="Reset All") -> (x .or. y?=w450:bool)
        n224 = local read "System Loop Type"() -> (w424:enum16{"Open Loop", "Closed Loop"})
        n225 = xnode "Read/Write Control"("FPGA VI Reference In"=w434, "error in"=w435, "Wait timer (ms)"="FPGA Wait Timer (ms)", "Controller Loop Period (uSec)"="Controller Time Period (uSec)", "Module Output Loop Period (uSec)"="Controller Output Time Period (uSec)", "System Loop Type"=w424, "Controller Output Upper Limit"="Controller Output Upper Limit", "Controller Output Lower Limit"="Controller Output Lower Limit", "X-Stage nm to V Scaling"="X-Stage nm to V Scaling", "X-Stage Scaling Direction"="X-Stage Scaling Direction", "Y-Stage nm to V Scaling"="Y-Stage nm to V Scaling", "Z-Stage nm to V Scaling"="Z-Stage nm to V Scaling", "Plant Output Loop Period (uSec)"="Plant Output Time Period (uSec)", "Reset Optics X"=w456, "Reset Optics Y"=w454, "Reset Optics Z"=w452, "Reset Sample X"=w451, "Reset Sample Y"=w450, "Reset Sample Z"=w449, "Optics X Stage Resolution (nm)"="Optics X Stage Resolution (nm)", "Optics Y Stage Resolution (nm)"="Optics Y Stage Resolution (nm)", "Optics Z Stage Resolution (nm)"="Optics Z Stage Resolution (nm)", "Sample X Stage Resolution (nm)"="Sample X Stage Resolution (nm)", "Sample Y Stage Resolution (nm)"="Sample Y Stage Resolution (nm)", "Sample Z Stage Resolution (nm)"="Sample Z Stage Resolution (nm)", "Scaling mV to V"="Scaling mV to V", "-a01(2) xx1"=w472, "-a02(2) xx1"=w471, "b01(2) xx1"=w470, "b02(2) xx1"=w469, "sos gain SF Controller xx1"=w468, "-a01(2) yy1"=w467, "-a02(2) yy1"=w466, "b01(2) yy1"=w465, "b02(2) yy1"=w464, "sos gain SF Controller yy1"=w463, "-a01(2) zz1"=w462, "-a02(2) zz1"=w458, "b01(2) zz1"=w459, "b02(2) zz1"=w460, "sos gain SF Controller zz1"=w461, "Optics and or Sample Stage"="Optics and or Sample Stage", "Y-Stage Scaling Direction"="Y-Stage Scaling Direction", "Z-Stage Scaling Direction"="Z-Stage Scaling Direction") -> ("FPGA VI Reference Out"=w432:refnum<k20>, "error out"=w431:errorcluster)
      }
      frame "Wait" {
        n226 = shared-variable ".\\Interloop communication.lvlib\\New Command"() -> (w490:bool, error out=w488:errorcluster)  [unwired: 1 in]
        n227 = case shown="True" w490 {
          tunnel: [w493 w495] -> w489
          tunnel: w488 -> [_ w499]
          tunnel: w486 -> [w492 w497]
          tunnel: [w492 w496] -> w485
          tunnel: w483 -> [_ w494]
          frame False {
            w493 = T9[] [enum."Wait"] items=["Initialization", "Import Controller coeffs", "Update Controller Info", "Wait", "Update Reference Info", "Update Detector Trigger Info", "Update Datalog Info", "Check FPGA Status", "Initialize FIFO", "Pre-Scan", "Start Scan", "Step Scanning", "Fly Scanning", "End Scan", "Close File", "Restart FPGA", "Stop FPGA"]
          }
          frame True {
            n228 = shared-variable ".\\Interloop communication.lvlib\\System command"() -> (w498:T6)  [unwired: 1 in, 1 out]
            "Last Command Executed" <- w498
            n229 = case shown="\"Scan\"" w498 {
              tunnel: [w503 w506 w510 w515 w518 w522] -> w495
              tunnel: w497 -> [w502 w505 w509 w514 w517 w521]
              tunnel: [w501 w504 w508 w513 w516 w520] -> w496
              tunnel: w494 -> [_ _ w507 _ _ _]
              frame "Re-Initialize ", Default {
                w503 = T9[] [enum."Initialization", enum."Import Controller coeffs", enum."Update Controller Info", enum."Wait"] items=["Initialization", "Import Controller coeffs", "Update Controller Info", "Wait", "Update Reference Info", "Update Detector Trigger Info", "Update Datalog Info", "Check FPGA Status", "Initialize FIFO", "Pre-Scan", "Start Scan", "Step Scanning", "Fly Scanning", "End Scan", "Close File", "Restart FPGA", "Stop FPGA"]
                n230 = call <vilib>:"Clear Errors.vi"("error in (no error)"=w502) -> ("error out"=w501:errorcluster)  [unwired: 5 in, 1 out]
              }
              frame "Update Scan Settings" {
                w506 = T9[] [enum."Update Reference Info", enum."Update Detector Trigger Info", enum."Update Datalog Info", enum."Wait"] items=["Initialization", "Import Controller coeffs", "Update Controller Info", "Wait", "Update Reference Info", "Update Detector Trigger Info", "Update Datalog Info", "Check FPGA Status", "Initialize FIFO", "Pre-Scan", "Start Scan", "Step Scanning", "Fly Scanning", "End Scan", "Close File", "Restart FPGA", "Stop FPGA"]
                n231 = call <vilib>:"Clear Errors.vi"("error in (no error)"=w505) -> ("error out"=w504:errorcluster)  [unwired: 5 in, 1 out]
              }
              frame "Scan" {
                n232 = case shown="\"Fly\", Default" w507 {
                  tunnel: [w511 w512] -> w510
                  frame "Fly", Default {
                    w511 = T9[] [enum."Update Reference Info", enum."Update Detector Trigger Info", enum."Update Datalog Info", enum."Pre-Scan", enum."Start Scan", enum."Fly Scanning", enum."End Scan", enum."Close File", enum."Wait"] items=["Initialization", "Import Controller coeffs", "Update Controller Info", "Wait", "Update Reference Info", "Update Detector Trigger Info", "Update Datalog Info", "Check FPGA Status", "Initialize FIFO", "Pre-Scan", "Start Scan", "Step Scanning", "Fly Scanning", "End Scan", "Close File", "Restart FPGA", "Stop FPGA"]
                  }
                  frame "Step" {
                    w512 = T9[] [enum."Update Reference Info", enum."Update Detector Trigger Info", enum."Update Datalog Info", enum."Pre-Scan", enum."Start Scan", enum."Step Scanning", enum."End Scan", enum."Wait"] items=["Initialization", "Import Controller coeffs", "Update Controller Info", "Wait", "Update Reference Info", "Update Detector Trigger Info", "Update Datalog Info", "Check FPGA Status", "Initialize FIFO", "Pre-Scan", "Start Scan", "Step Scanning", "Fly Scanning", "End Scan", "Close File", "Restart FPGA", "Stop FPGA"]
                  }
                }
                n233 = call <vilib>:"Clear Errors.vi"("error in (no error)"=w509) -> ("error out"=w508:errorcluster)  [unwired: 5 in, 1 out]
              }
              frame "Stop Scan" {
                w515 = T9[] [enum."End Scan", enum."Wait"] items=["Initialization", "Import Controller coeffs", "Update Controller Info", "Wait", "Update Reference Info", "Update Detector Trigger Info", "Update Datalog Info", "Check FPGA Status", "Initialize FIFO", "Pre-Scan", "Start Scan", "Step Scanning", "Fly Scanning", "End Scan", "Close File", "Restart FPGA", "Stop FPGA"]
                n234 = call <vilib>:"Clear Errors.vi"("error in (no error)"=w514) -> ("error out"=w513:errorcluster)  [unwired: 5 in, 1 out]
              }
              frame "Restart FPGA" {
                w518 = T9[] [enum."Restart FPGA", enum."Initialization", enum."Import Controller coeffs", enum."Update Controller Info", enum."Wait"] items=["Initialization", "Import Controller coeffs", "Update Controller Info", "Wait", "Update Reference Info", "Update Detector Trigger Info", "Update Datalog Info", "Check FPGA Status", "Initialize FIFO", "Pre-Scan", "Start Scan", "Step Scanning", "Fly Scanning", "End Scan", "Close File", "Restart FPGA", "Stop FPGA"]
                n235 = call <vilib>:"Clear Errors.vi"("error in (no error)"=w517) -> ("error out"=w516:errorcluster)  [unwired: 5 in, 1 out]
              }
              frame "Stop System" {
                w522 = T9[] [enum."Stop FPGA"] items=["Initialization", "Import Controller coeffs", "Update Controller Info", "Wait", "Update Reference Info", "Update Detector Trigger Info", "Update Datalog Info", "Check FPGA Status", "Initialize FIFO", "Pre-Scan", "Start Scan", "Step Scanning", "Fly Scanning", "End Scan", "Close File", "Restart FPGA", "Stop FPGA"]
                n236 = call <vilib>:"Clear Errors.vi"("error in (no error)"=w521) -> ("error out"=w520:errorcluster)  [unwired: 5 in, 1 out]
                n237 = shared-variable ".\\Interloop communication.lvlib\\Stop System"(TRUE ("Stop")) -> ()  [unwired: 1 in, 1 out]
              }
            }
            n238 = shared-variable ".\\Interloop communication.lvlib\\New Command"(FALSE ("New Command"), error in=w499) -> ()  [unwired: 1 out]
          }
        }
      }
      frame "Update Reference Info" {
        w551 = 40000000.0  # FPGA clock rate (Hz)
        n239 = shared-variable ".\\Interloop communication.lvlib\\X Ramp Start (nm)"() -> (w531:fxp<+/-,32,16>)  [unwired: 1 in, 1 out]
        n240 = shared-variable ".\\Interloop communication.lvlib\\Y Ramp Start (nm)"() -> (w533:fxp<+/-,32,16>)  [unwired: 1 in, 1 out]
        n241 = shared-variable ".\\Interloop communication.lvlib\\Rotation Direction"() -> (w529:enum16{"Clockwise", "Anti-clockwise"})  [unwired: 1 in, 1 out]
        n242 = shared-variable ".\\Interloop communication.lvlib\\X Ramp End (nm)"() -> (w532:fxp<+/-,32,16>)  [unwired: 1 in, 1 out]
        n243 = shared-variable ".\\Interloop communication.lvlib\\Y Ramp End (nm)"() -> (w534:fxp<+/-,32,16>)  [unwired: 1 in, 1 out]
        n244 = shared-variable ".\\Interloop communication.lvlib\\X Step Size (nm)"() -> (w535:fxp<+/-,32,16>)  [unwired: 1 in, 1 out]
        n245 = shared-variable ".\\Interloop communication.lvlib\\Y Step Size (nm)"() -> (w527:fxp<+/-,32,16>)  [unwired: 1 in, 1 out]
        n246 = shared-variable ".\\Interloop communication.lvlib\\Radial direction"() -> (w528:enum16{"Outward", "Inward"})  [unwired: 1 in, 1 out]
        n247 = shared-variable ".\\Interloop communication.lvlib\\Spiral Step Size"() -> (w525:fxp<+/-,32,16>)  [unwired: 1 in, 1 out]
        n248 = shared-variable ".\\Interloop communication.lvlib\\Inner Scan axis"() -> (w530:enum16{"X", "Y"})  [unwired: 1 in, 1 out]
        n249 = shared-variable ".\\Interloop communication.lvlib\\Max radius"() -> (w526:fxp<+/-,32,16>)  [unwired: 1 in, 1 out]
        n250 = call <vilib>:"Normalize Signal Generation Parameters.vi"("frequency (Hz)"="Trajectory frequency (Hz)", "FPGA clock rate (Hz)"=w551, "error in (no error)"=w540) -> ("frequency (periods/tick)"=w542:fxp<+,32,0>, "actual frequency (Hz)"=→"actual Traj frequency (Hz)":dbl, "error out"=w539:errorcluster)  [unwired: 7 in, 3 out]
        "Trajectory frequency (periods/tick)" <- w542
        n251 = local read "Scan Geometry"() -> (w524:T3)
        n252 = xnode "Read/Write Control"("FPGA VI Reference In"=w548, "error in"=w539, "XY Reference Loop Period (us)"="XY Reference Time Period (uSec)", "Z Reference Loop Period (us)"="Z Reference Time Period (uSec)", "Scan Geometry"=w524, "X Reference Amplitude (nm)"="X Reference Amplitude (nm)", "Y Reference Amplitude (nm)"="Y Reference Amplitude (nm)", "Z Reference Amplitude (nm)"="Z Reference Amplitude (nm)", "Traj Frequency"=w542, "X Reference DC Offset (nm)"="X Reference DC Offset (nm)", "Y Reference DC Offset (nm)"="Y Reference DC Offset (nm)", "Z Reference DC Offset (nm)"="Z Reference DC Offset (nm)", "Scan type"=w538, "Inner Scan axis"=w530, "Spiral Rotation Direction"=w529, "Radial direction"=w528, "X Start (nm)"=w531, "X End (nm)"=w532, "X Step Size"=w535, "Y Start (nm)"=w533, "Y End (nm)"=w534, "Y Step Size"=w527, "Max radius"=w526, "Spiral Step Size"=w525) -> ("FPGA VI Reference Out"=w546:refnum<k20>, "error out"=w545:errorcluster)
      }
      frame "Update Detector Trigger Info" {
        w562 = 40000000.0  # FPGA clock rate (Hz)
        w581 = 40000000.0  # FPGA clock rate (Hz)
        n253 = shared-variable ".\\Interloop communication.lvlib\\Det Frequency (Hz)"() -> (w568:dbl)  [unwired: 1 in, 1 out]
        "Det Trigger Frequency (Hz)" <- w568
        n254 = shared-variable ".\\Interloop communication.lvlib\\Det duty cycle (%)"() -> (w567:dbl)  [unwired: 1 in, 1 out]
        "Det Trigger Duty Cycle (%)" <- w567
        n255 = call <vilib>:"Normalize Signal Generation Parameters.vi"("frequency (Hz)"=w568, "FPGA clock rate (Hz)"=w581, "phase offset (deg)"="Det phase offset (deg)", "duty cycle (%)"=w567, "error in (no error)"=w570) -> ("frequency (periods/tick)"=w580:fxp<+,32,0>, "phase offset (periods)"=w579:fxp<+,32,0>, "duty cycle (periods)"=w578:fxp<+,32,0>, "error out"=w569:errorcluster)  [unwired: 5 in, 2 out]
        "Det Frequency (periods/tick)" <- w580
        "Det Phase Offset (periods)" <- w579
        "Det Duty Cycle (periods)" <- w578
        n256 = shared-variable ".\\Interloop communication.lvlib\\Data frequency (Hz)"() -> (w561:dbl)  [unwired: 1 in, 1 out]
        n257 = shared-variable ".\\Interloop communication.lvlib\\Data duty cycle (%)"() -> (w559:dbl)  [unwired: 1 in, 1 out]
        n258 = call <vilib>:"Normalize Signal Generation Parameters.vi"("frequency (Hz)"=w561, "FPGA clock rate (Hz)"=w562, "phase offset (deg)"="Data phase offset (deg)", "duty cycle (%)"=w559) -> ("frequency (periods/tick)"=w565:fxp<+,32,0>, "phase offset (periods)"=w564:fxp<+,32,0>, "duty cycle (periods)"=w563:fxp<+,32,0>)  [unwired: 6 in, 3 out]
        "Data Frequency" <- w565
        "Data Duty Cycle (periods)" <- w563
        "Data Phase Offset (periods)" <- w564
        n259 = xnode "Read/Write Control"("FPGA VI Reference In"=w577, "error in"=w569, "Trigger Generation Time Period (uSec)"="Trigger Generation Time Period (uSec)", "Detector Trigger Lower Limit (V)"="Detector Trigger Lower Limit (V)", "Detector Trigger Upper Limit (V)"="Detector Trigger Upper Limit (V)", "DT Reference Amplitude (V)"="Det Reference Amplitude (V)", "DT Reference DC Offset (V)"="DT Reference DC Offset (V)", "Det Frequency"=w580, "Det Phase Offset (periods)"=w579, "DT Reset"="Det Reset", "Det Duty Cycle (periods)"=w578, "Data Trigger Reset"="Data Trigger Reset", "Data Frequency"=w565, "Data Phase Offset (periods)"=w564, "Data Duty Cycle (periods)"=w563) -> ("FPGA VI Reference Out"=w575:refnum<k20>, "error out"=w574:errorcluster)
      }
      frame "Update Datalog Info" {
        n260 = xnode "Read/Write Control"("FPGA VI Reference In"=w599, "error in"=w598, "FIFO Loop Period (us)"="Datalog Time Period (uSec)", "Datalog Cases"="Datalog Cases", "Timeout FPGA FIFO1"="Timeout FPGA FIFO1") -> ("FPGA VI Reference Out"=w596:refnum<k20>, "error out"=w595:errorcluster)
      }
      frame "Check FPGA Status" {
        n261 = xnode "Read/Write Control"("FPGA VI Reference In"=w614, "error in"=w613) -> ("FPGA VI Reference Out"=w612:refnum<k20>, "error out"=w611:errorcluster, "FPGA error monitor"=w617:errorcluster, "End Run Error"=w616:errorcluster, "FIFO Timed Out?"=→"FIFO Timed Out?":bool, "Stop Scan"=w606:bool, "FIFO Timed Out"=w607:bool)
        "FPGA end run error" <- w616
        "Stop Run" <- w606
        "FIFO Timed Out" <- w607
        n262 = case shown="True" w606 {
          tunnel: [errorcluster {"status"=FALSE, "code"=0, "source"=""} ("error constant") errorcluster {"status"=TRUE, "code"=7002, "source"="FPGA stop case encountered"} ("error constant")] -> w604
          frame False {
          }
          frame True {
          }
        }
        n263 = case shown="True" w607 {
          tunnel: [errorcluster {"status"=FALSE, "code"=0, "source"=""} ("error constant") errorcluster {"status"=TRUE, "code"=7001, "source"="FPGA FIFO timed out"} ("error constant")] -> w605
          frame False {
          }
          frame True {
          }
        }
        n264 = Merge Errors(w611, w617, w616, w604, w605) -> (w603:errorcluster)
      }
      frame "Pre-Scan" {
        n265 = flat-sequence {
          tunnel: w635 -> [w649]
          tunnel: w634 -> [w648]
          tunnel: [w645] -> w633
          tunnel: [w644] -> w631
          tunnel: w633 -> [w652]
          tunnel: [w652] -> w632
          tunnel: w631 -> [w651]
          tunnel: [w651] -> w630
          tunnel: w632 -> [w656]
          tunnel: w630 -> [w655]
          tunnel: [w654] -> w629
          tunnel: [w653] -> w628
          tunnel: w629 -> [w665]
          tunnel: w628 -> [w664]
          tunnel: w625 -> [w660]
          tunnel: [w659] -> w624
          tunnel: [w658] -> w623
          frame #0 {
            w639 = fxp<+/-,16,16> 0.0
            w646 = TRUE
            n266 = xnode "Read/Write Control"("FPGA VI Reference In"=w649, "error in"=w648, "Reset Optics X"=w646, "Reset Optics Y"=w646, "Reset Optics Z"=w646, "Reset Sample X"=w646, "Reset Sample Y"=w646, "Reset Sample Z"=w646, "System Loop Type"=enum16{"Open Loop", "Closed Loop"}."Open Loop", "Data Save Flag"=enum16{"Skip Data", "Save Data"}."Skip Data", "Scan type"=enum16{"Fly", "Step"}."Step", "FPGA command"=enum16{"Start Scan", "Shutdown"}."Start Scan", "X Reference Amplitude (nm)"="X Start Marker (nm)", "Y Reference Amplitude (nm)"="Y Start Marker (nm)", "X Reference DC Offset (nm)"=w639, "Y Reference Amplitude (nm)"=w639, "New FPGA command"=TRUE) -> ("FPGA VI Reference Out"=w645:refnum<k20>, "error out"=w644:errorcluster)
          }
          frame #1 {
            n267 = Wait (ms)(milliseconds to wait="Pre-Scan pause (ms)") -> ()  [unwired: 1 out]
          }
          frame #2 {
            n268 = xnode ("Read/Write Control")("FPGA VI Reference In"=w656, "error in"=w655, "Stop Scan"=TRUE ("stop case")) -> ("FPGA VI Reference Out"=w654:refnum<k20>, "error out"=w653:errorcluster)
          }
          frame #3 {
            w662 = FALSE ("Reset Optics X")
            n269 = local read "System Loop Type"() -> (w663:enum16{"Open Loop", "Closed Loop"})
            n270 = xnode "Read/Write Control"("FPGA VI Reference In"=w665, "error in"=w664, "Reset Optics X"=w662, "Reset Optics Y"=w662, "Reset Optics Z"=w662, "Reset Sample X"=w662, "Reset Sample Y"=w662, "Reset Sample Z"=w662, "System Loop Type"=w663, "Data Save Flag"="Data Save Flag", "Scan type"=w660) -> ("FPGA VI Reference Out"=w659:refnum<k20>, "error out"=w658:errorcluster)
          }
        }
      }
      frame "Start Scan" {
        n271 = case shown="\"Fly\", Default" w679 {
          tunnel: w680 -> [w688 w703]
          tunnel: w666 -> [w693 w704]
          tunnel: [w692 w704] -> w669
          tunnel: [w689 w703] -> w670
          frame "Fly", Default {
            n272 = xnode ("Invoke Method")("FPGA VI Reference In"=w693, "error in"=w688, "Requested Depth"="Requested Depth") -> ("FPGA VI Reference Out"=w687:refnum<k20>, "error out"=w686:errorcluster, "Actual Depth"=→"Actual Depth":u32)
            n273 = shared-variable ".\\Interloop communication.lvlib\\Base Filename"() -> (w696:string)  [unwired: 1 in, 1 out]
            n274 = call "Clear FPGA FIFO.vi"("error in (no error)"=w686, "Refnum in"=w687) -> ("error out"=w683:errorcluster, "Data"=→"Cleared Data":fxp<+/-,40,32>[], "Refnum out"=w684:refnum<k20>)  [unwired: 7 in]
            n275 = String To Path(string="cRIO data dir") -> (path=w697:path)
            "cRIO path" <- w697
            n276 = xnode "Invoke Method"("FPGA VI Reference In"=w684, "error in"=w683) -> ("FPGA VI Reference Out"=w692:refnum<k20>, "error out"=w691:errorcluster)
            n277 = call "Data_Write.vi"("Destination dir"=w697, "error initialize"=w688, "Base name"=w696, "Command List"=Data_Write_Control."Initialize") -> ("error out"=w690:errorcluster, "Path"=w701:path)  [unwired: 4 in]
            n278 = Strip Path(path=w701) -> (stripped path=→"Output path":path, name=→"Output filename":string)
            n279 = Merge Errors(w691, w690) -> (w689:errorcluster)
          }
          frame "Step" {
          }
        }
        n280 = xnode "Read/Write Control"("FPGA VI Reference In"=w669, "error in"=w670) -> ("FPGA VI Reference Out"=w672:refnum<k20>, "error out"=w673:errorcluster, "Trajectory Complete"=w671:bool)
        n281 = xnode "Read/Write Control"("FPGA VI Reference In"=w672, "error in"=w673, "New FPGA command"=TRUE, "FPGA command"=enum16{"Start Scan", "Shutdown"}."Start Scan") -> ("FPGA VI Reference Out"=w677:refnum<k20>, "error out"=w676:errorcluster)
        n282 = local write "Trajectory Completed"(w671) -> ()
      }
      frame "Step Scanning" {
        n283 = shared-variable ".\\Interloop communication.lvlib\\Y Reference Amplitude (nm)"() -> (w707:fxp<+/-,40,17>)  [unwired: 1 in, 1 out]
        n284 = shared-variable ".\\Interloop communication.lvlib\\Z Reference Amplitude (nm)"() -> (w706:fxp<+/-,40,17>)  [unwired: 1 in, 1 out]
        n285 = shared-variable ".\\Interloop communication.lvlib\\X Reference Amplitude (nm)"() -> (w708:fxp<+/-,40,17>)  [unwired: 1 in, 1 out]
        n286 = Insert Into Array(array=w719, index=0, new element=State_Enum."Step Scanning" ("new element/subarray")) -> (w718:T9[])
        n287 = xnode "Read/Write Control"("FPGA VI Reference In"=w713, "error in"=w712, "X Reference Amplitude (nm)"=w708, "Y Reference Amplitude (nm)"=w707, "Z Reference Amplitude (nm)"=w706) -> ("FPGA VI Reference Out"=w711:refnum<k20>, "error out"=w710:errorcluster)
      }
      frame "Fly Scanning" {
        n288 = xnode "Read/Write Control"("FPGA VI Reference In"=w748, "error in"=w729) -> ("FPGA VI Reference Out"=w743:refnum<k20>, "error out"=w742:errorcluster, "FPGA state"=w738:T12)
        n289 = Equal?(x=T12."Wait", y=w738) -> (x = y?=w735:bool)
        n290 = xnode "Invoke Method"("FPGA VI Reference In"=w743, "error in"=w742, "Number of Elements"=u32 0, "Timeout (ms)"=100) -> ("FPGA VI Reference Out"=w740:refnum<k20>, "error out"=w741:errorcluster, "Elements Remaining"=w724:u32)  [unwired: 1 out]
        "Elements Available in FIFO" <- w724
        n291 = Equal?(x=u32 0, y=w724) -> (x = y?=w736:bool)
        n292 = Compound Arithmetic op=AND(w722, w735, w736) -> (w734:bool)
        n293 = case shown="False" w734 {
          tunnel: w733 -> [w753 w754]
          tunnel: [w751 w754] -> w732
          frame False {
            # "Either FIFO not empty or FPGA not \ndone running -- repeat scanning state"
            n294 = Insert Into Array(array=w753, index=0, new element=State_Enum."Fly Scanning" ("new element/subarray")) -> (w751:T9[])
          }
          frame True {
            # "FIFO empty, FPGA done running \n-- moving onto next state"
          }
        }
        n295 = xnode ("Invoke Method")("FPGA VI Reference In"=w740, "error in"=w741, "Number of Elements"=w724, "Timeout (ms)"="FIFO Timeout (ms)") -> ("FPGA VI Reference Out"=w726:refnum<k20>, "error out"=w747:errorcluster, "Data"=w730:fxp<+/-,40,32>[], "Elements Remaining"=→"Elements Remaining" →"Elements Remaining in FIFO":u32)
        "Data" <- w730
        n296 = Enqueue Element(queue=w727, element=w730, error in (no error)=w729) -> (error out=w728:errorcluster)  [unwired: 1 in, 2 out]
        n297 = Merge Errors(w747, w728) -> (w746:errorcluster)
      }
      frame "End Scan" {
        n298 = case shown="\"Fly\", Default" w766 {
          tunnel: w770 -> [w795 w796]
          tunnel: [w794 w796] -> w769
          tunnel: w768 -> [w793 w797]
          tunnel: [w792 w797] -> w767
          frame "Fly", Default {
            n299 = xnode "Invoke Method"("FPGA VI Reference In"=w795, "error in"=w793) -> ("FPGA VI Reference Out"=w794:refnum<k20>, "error out"=w792:errorcluster)
          }
          frame "Step" {
          }
        }
        n300 = xnode "Read/Write Control"("FPGA VI Reference In"=w769, "error in"=w767, "Stop Scan"=TRUE ("New FPGA command")) -> ("FPGA VI Reference Out"=w759:refnum<k20>, "error out"=w758:errorcluster)
        n301 = flat-sequence {
          tunnel: w759 -> [w783]
          tunnel: w758 -> [w782]
          tunnel: [w780] -> w763
          tunnel: [w779] -> w762
          tunnel: w763 -> [w786]
          tunnel: [w786] -> w761
          tunnel: w762 -> [w785]
          tunnel: [w785] -> w760
          tunnel: w761 -> [w790]
          tunnel: w760 -> [w789]
          tunnel: [w788] -> w757
          tunnel: [w787] -> w756
          frame #0 {
            w778 = fxp<+/-,40,17> 0.0 ("Y Reference Amplitude (nm)")
            n302 = xnode "Read/Write Control"("FPGA VI Reference In"=w783, "error in"=w782, "System Loop Type"=enum16{"Open Loop", "Closed Loop"}."Open Loop", "FPGA command"=enum16{"Start Scan", "Shutdown"}."Start Scan", "Data Save Flag"=enum16{"Skip Data", "Save Data"}."Skip Data", "Scan type"=enum16{"Fly", "Step"}."Step", "X Reference Amplitude (nm)"=w778, "Y Reference Amplitude (nm)"=w778, "New FPGA command"=TRUE) -> ("FPGA VI Reference Out"=w780:refnum<k20>, "error out"=w779:errorcluster)
          }
          frame #1 {
            n303 = Wait (ms)(milliseconds to wait="Post-Scan pause (ms)") -> ()  [unwired: 1 out]
          }
          frame #2 {
            n304 = xnode ("Read/Write Control")("FPGA VI Reference In"=w790, "error in"=w789, "Stop Scan"=TRUE ("stop case")) -> ("FPGA VI Reference Out"=w788:refnum<k20>, "error out"=w787:errorcluster)
          }
        }
      }
      frame "Close File" {
        n305 = local read "Queue is empty"() -> (w801:bool)
        n306 = case shown="True" w801 {
          tunnel: w804 -> [w809 w818]
          tunnel: w806 -> [w811 w816]
          tunnel: [w810 w816] -> w807
          tunnel: [w809 w815] -> w798
          tunnel: [TRUE FALSE] -> w799
          frame False {
            # "Queue is not empty, so file is still be written to"
            n307 = Insert Into Array(array=w811, index=0, new element=State_Enum."Close File" ("new element/subarray")) -> (w810:T9[])
          }
          frame True {
            n308 = call "Data_Write.vi"("error initialize"=w818, "Command List"=Data_Write_Control."Close") -> ("error out"=w817:errorcluster)  [unwired: 6 in, 1 out]
            n309 = case shown="No Error" w817 {
              tunnel: w817 -> [w825 w826]
              tunnel: [w824 w826] -> w815
              frame No Error {
                n310 = local read "Output filename"() -> (w820:string)
                n311 = local read "Output path"() -> (w821:path)
                n312 = Path To String(path=w821) -> (string=w823:string)
                n313 = shared-variable "RT CompactRIO Target\\RT_EPICS_Shared_Variables.lvlib\\2iddVELO:VP:Last_Filename"(w820, error in=w825) -> (error out=w822:errorcluster)
                n314 = shared-variable "RT CompactRIO Target\\RT_EPICS_Shared_Variables.lvlib\\2iddVELO:VP:cRIO_Dir"(w823, error in=w822) -> (error out=w824:errorcluster)
              }
              frame Error {
              }
            }
          }
        }
      }
      frame "Restart FPGA" {
        n315 = call <vilib>:"Clear Errors.vi"("error in (no error)"=w835) -> ("error out"=w836:errorcluster)  [unwired: 5 in, 1 out]
        n316 = xnode "Invoke Method"("FPGA VI Reference In"=w841, "error in"=w836) -> ("FPGA VI Reference Out"=w840:refnum<k20>, "error out"=w839:errorcluster)
        n317 = shared-variable "RT CompactRIO Target\\RT_EPICS_Shared_Variables.lvlib\\2iddVELO:VP:Scanning"(FALSE ("2iddVELO:VP:Scanning")) -> ()  [unwired: 1 in, 1 out]
        n318 = xnode "Read/Write Control"("FPGA VI Reference In"=w840, "error in"=w839, "Stop Scan"=TRUE ("stop case")) -> ("FPGA VI Reference Out"=w834:refnum<k20>, "error out"=w833:errorcluster)
        n319 = xnode "Invoke Method"("FPGA VI Reference In"=w834, "error in"=w833) -> ("FPGA VI Reference Out"=w832:refnum<k20>, "error out"=w831:errorcluster)
      }
      frame "Stop FPGA" {
        w852 = T9[] [enum."Stop FPGA"] items=["Initialization", "Import Controller coeffs", "Update Controller Info", "Wait", "Update Reference Info", "Update Detector Trigger Info", "Update Datalog Info", "Check FPGA Status", "Initialize FIFO", "Pre-Scan", "Start Scan", "Step Scanning", "Fly Scanning", "End Scan", "Close File", "Restart FPGA", "Stop FPGA"] ("Reduced Array of States")
        w851 = TRUE ("stop case")
        n320 = xnode "Invoke Method"("FPGA VI Reference In"=w859, "error in"=w858) -> ("FPGA VI Reference Out"=w857:refnum<k20>, "error out"=w856:errorcluster)
        n321 = shared-variable "RT CompactRIO Target\\RT_EPICS_Shared_Variables.lvlib\\2iddVELO:VP:Scanning"(FALSE ("2iddVELO:VP:Scanning")) -> ()  [unwired: 1 in, 1 out]
        n322 = xnode "Read/Write Control"("FPGA VI Reference In"=w857, "error in"=w856, "Stop Scan"=w851, "New FPGA command"=w851, "FPGA command"=enum16{"Start Scan", "Shutdown"}."Shutdown") -> ("FPGA VI Reference Out"=w855:refnum<k20>, "error out"=w848:errorcluster)
        n323 = xnode "Invoke Method"("FPGA VI Reference In"=w855, "error in"=w848) -> ("FPGA VI Reference Out"=w849:refnum<k20>, "error out"=w847:errorcluster)
        n324 = xnode "Close FPGA VI Reference"("FPGA VI Reference In"=w849, "error in"=w847) -> ("error out"=w854:errorcluster)
      }
    }
    "Main Loop error" <- w358
    n325 = Format Into String(format string="%s", w354) -> (resulting string=w355:string)  [unwired: 2 in, 1 out]
    n326 = shared-variable "RT CompactRIO Target\\RT_EPICS_Shared_Variables.lvlib\\2iddVELO:VP:RT_State"(w355) -> ()  [unwired: 1 in, 1 out]
    n327 = shared-variable "RT CompactRIO Target\\RT_EPICS_Shared_Variables.lvlib\\2iddVELO:VP:Scanning"(w347) -> ()  [unwired: 1 in, 1 out]
    n328 = shared-variable ".\\Interloop communication.lvlib\\Main Loop Error"(w358) -> ()  [unwired: 1 in, 1 out]
    n329 = node-c288(w361) -> ()  [unwired: 1 out]
    n330 = call "State Control.vi"("Stop"=FALSE, "Array of States"=w366, "Error Input"=w358) -> ("Next State"=w348:T9, "Reduced Array of States"=w362:T9[])  [unwired: 5 in]
    "RT Main Loop State" <- w354
    "Main Loop Iterations" <- w364
    "Reduced Array of States" <- w363
  }
  n331 = while {
    tunnel: w11 -> [w883]
    shift-right: [w870] -> _
    shift-left: _ -> [w869]
    tunnel: w9 -> [w867]
    tunnel: w3 -> [w865]
    i -> [w876]
    stop <- w877 stop-if-true
    # "Data writing and plotting loop"
    n332 = Get Queue Status(queue=w883, error in (no error)=w867) -> (queue out=w881:refnum<queue>, error out=w882:errorcluster, # elements in queue=w879:i32)  [unwired: 1 in, 5 out]
    n333 = Greater Than 0?(x=w879) -> (x > 0?=w880:bool)
    n334 = case shown="True" w880 {
      tunnel: w882 -> [w890 w916]
      tunnel: w881 -> [_ w915]
      tunnel: [w890 w896] -> w866
      tunnel: [TRUE FALSE] -> w875
      tunnel: [w884 w910] -> w870
      tunnel: w869 -> [w886 w909]
      tunnel: w865 -> [_ w892]
      frame False {
        n335 = local read "RT Main Loop State"() -> (w889:T9)
        n336 = Equal?(x=w889, y=State_Enum."Fly Scanning") -> (x = y?=w887:bool)
        n337 = Select(t=w886, s=w887, f=fxp<+/-,58,25>[] []) -> (s? t:f=w884:fxp<+/-,58,25>[])
      }
      frame True {
        w918 = "%8f"  # format string
        w919 = ","  # delimiter (Tab)
        n338 = shared-variable ".\\Interloop communication.lvlib\\Data frequency (Hz)"() -> (w895:dbl)  [unwired: 1 in, 1 out]
        n339 = Dequeue Element(queue=w915, error in (no error)=w916) -> (element=w903:fxp<+/-,58,25>[], error out=w914:errorcluster)  [unwired: 1 in, 2 out]
        n340 = Decimate 1D Array(w903) -> (w908:fxp<+/-,58,25>[], w907:fxp<+/-,58,25>[], w906:fxp<+/-,58,25>[], w905:fxp<+/-,58,25>[], w904:fxp<+/-,58,25>[])
        n341 = Build Array(w908, w907, w906, w905, w904) -> (w902:fxp<+/-,58,25>[][])
        n342 = case shown="\"Partial Plot\"" "Plot option" {
          tunnel: [fxp<+/-,58,25>[] [] fxp<+/-,58,25>[] [] w957] -> w910
          tunnel: w909 -> [_ _ w956]
          tunnel: w903 -> [_ w927 w953]
          tunnel: [cluster{dbl[], dbl[]}[] [] w931 w951] -> w900
          tunnel: [cluster{"t0":dbl, dbl, dbl[][]} {"t0"=0.0, 0.0, []} w930 w950] -> w899
          tunnel: [w922 w929 w949] -> w898
          tunnel: w895 -> [w921 w928 w948]
          tunnel: [w921 w928 w948] -> w897
          frame "No Plot", Default {
            n343 = Reciprocal(x=w921) -> (1/x=w922:dbl)
          }
          frame "Partial Plot" {
            w939 = 0.0  # t0
            n344 = Decimate 1D Array(w927) -> (w942:fxp<+/-,58,25>[], w943:fxp<+/-,58,25>[], w944:fxp<+/-,58,25>[], w945:fxp<+/-,58,25>[], w941:fxp<+/-,58,25>[])
            n345 = Build Array(w942, w943, w944, w945, w941) -> (w940:fxp<+/-,58,25>[][])
            n346 = To Double Precision Float(number=w942) -> (double precision float=w937:dbl[])
            n347 = To Double Precision Float(number=w943) -> (double precision float=w936:dbl[])
            n348 = To Double Precision Float(number=w944) -> (double precision float=w935:dbl[])
            n349 = To Double Precision Float(number=w945) -> (double precision float=w934:dbl[])
            n350 = Reciprocal(x=w928) -> (1/x=w929:dbl)
            n351 = To Double Precision Float(number=w940) -> (double precision float=w932:dbl[][])
            n352 = Bundle(w935, w934) -> (w933:cluster{dbl[], dbl[]})  [unwired: 1 in]
            n353 = Bundle(w937, w936) -> (w938:cluster{dbl[], dbl[]})  [unwired: 1 in]
            n354 = Build Array(w938, w933) -> (w931:cluster{dbl[], dbl[]}[])
            n355 = Bundle("t0"=w939, w929, w932) -> (w930:cluster{"t0":dbl, dbl, dbl[][]})  [unwired: 1 in]
          }
          frame "Full Plot" {
            w963 = 0.0  # t0
            n356 = Array Size(array=w956) -> (size(s)=w955:i32)
            n357 = Insert Into Array(array=w956, index=w955, new element=w953) -> (w957:fxp<+/-,58,25>[])
            n358 = Decimate 1D Array(w957) -> (w966:fxp<+/-,58,25>[], w967:fxp<+/-,58,25>[], w968:fxp<+/-,58,25>[], w969:fxp<+/-,58,25>[], w965:fxp<+/-,58,25>[])
            n359 = Reciprocal(x=w948) -> (1/x=w949:dbl)
            n360 = To Double Precision Float(number=w966) -> (double precision float=w961:dbl[])
            n361 = To Double Precision Float(number=w967) -> (double precision float=w960:dbl[])
            n362 = To Double Precision Float(number=w968) -> (double precision float=w959:dbl[])
            n363 = To Double Precision Float(number=w969) -> (double precision float=w958:dbl[])
            n364 = Build Array(w966, w967, w968, w969, w965) -> (w964:fxp<+/-,58,25>[][])
            n365 = Multiply(x=w949, y=1000.0) -> (x*y=w947:dbl)
            n366 = To Double Precision Float(number=w964) -> (double precision float=w952:dbl[][])
            n367 = Bundle(w959, w958) -> (w954:cluster{dbl[], dbl[]})  [unwired: 1 in]
            n368 = Bundle(w961, w960) -> (w962:cluster{dbl[], dbl[]})  [unwired: 1 in]
            n369 = Bundle("t0"=w963, w947, w952) -> (w950:cluster{"t0":dbl, dbl, dbl[][]})  [unwired: 1 in]
            n370 = Build Array(w962, w954) -> (w951:cluster{dbl[], dbl[]}[])
          }
        }
        "XY Ref" <- w900
        "Reference and Actual positions" <- w899
        "Data Read Period (sec)" <- w898
        "Data Read Rate (Hz)" <- w897
        n371 = To Double Precision Float(number=w902) -> (double precision float=w894:dbl[][])
        n372 = Enqueue Element(queue=w892, element=w894) -> (error out=w893:errorcluster)  [unwired: 2 in, 2 out]
        n373 = Transpose 2D Array(2D array=w894) -> (transposed array=w912:dbl[][])
        n374 = Array To Spreadsheet String(delimiter (Tab)=w919, array=w912, 3:w918) -> (spreadsheet string=w920:string)
        n375 = call "Data_Write.vi"("error initialize"=w914, "Data"=w920, "Command List"=Data_Write_Control."Write") -> ("error out"=w913:errorcluster)  [unwired: 5 in, 1 out]
        n376 = Merge Errors(w893, w913) -> (w896:errorcluster)
      }
    }
    "Queue is empty" <- w875
    "File Writer loop error" <- w866
    n377 = shared-variable ".\\Interloop communication.lvlib\\Stop System"() -> (w868:bool)  [unwired: 1 in, 1 out]
    n378 = Equal To 0?(x=w879) -> (x = 0?=w878:bool)
    n379 = local read "Fly scan loop dt"() -> (w872:i64)
    n380 = shared-variable ".\\Interloop communication.lvlib\\Data writer loop"(w866) -> ()  [unwired: 1 in, 1 out]
    n381 = And(x=w868, y=w878) -> (x .and. y?=w877:bool)
    n382 = Divide(x=w872, y=i64 2) -> (x/y=w873:dbl)
    n383 = To Unsigned Long Integer(number=w873) -> (unsigned 32bit integer=w871:u32)
    n384 = Wait Until Next ms Multiple(millisecond multiple=w871) -> ()  [unwired: 1 out]
    "File writer loop iterations" <- w876
  }
  n385 = while {
    tunnel: w10 -> [w974]
    tunnel: w16 -> [w973]
    i -> [w972]
    stop <- w970 stop-if-true
    # "Readback loop"
    n386 = local read "RT Main Loop State"() -> (w977:T9)
    n387 = Not Equal?(x=w977, y=State_Enum."Initialization") -> (x != y?=w975:bool)
    n388 = case shown="True" w975 {
      tunnel: w974 -> [_ w1020]
      tunnel: w973 -> [_ w1019]
      tunnel: [u32 100 ("milliseconds to wait") "Readback Loop time between iterations (ms)"] -> w971
      frame False {
      }
      frame True {
        w1043 = 40000000.0  # FPGA Clock Rate (Hz)
        w990 = 40000000.0  # FPGA Clock Rate (Hz)
        w1060 = 40000000.0  # FPGA Clock Rate (Hz)
        n389 = xnode "Read/Write Control"("FPGA VI Reference In"=w1020, "error in"=w1019) -> ("FPGA VI Reference Out"=w1010:refnum<k20>, "error out"=w1011:errorcluster, "FPGA state"=w1016:T12, "Trajectory Complete"=→"Trajectory Completed":bool, "Run Loop error"=→"FPGA Run Loop error":errorcluster, "FPGA error monitor"=→"FPGA error monitor":errorcluster, "Stop Scan"=w986:bool)
        "FPGA state" <- w1016
        n390 = local write "Stop Run"(w986) -> ()
        n391 = Format Into String(format string="%s", w1016) -> (resulting string=w1018:string)  [unwired: 2 in, 1 out]
        n392 = xnode ("Read/Write Control")("FPGA VI Reference In"=w1010, "error in"=w1011) -> ("error out"=w1015:errorcluster, "Detector Trigger In Range?"=→"Detector Trigger In Range?":bool, "Number of Data Strings"=→"Number of Data Strings":i32, "Scan Type and Geometry"=→"Scan Type and Geometry":T10, "Position Number"=→"Position Number":u32, "Controller Output Lower Limit"=→"Controller Output Lower Limit Readback":fxp<+/-,20,5>, "Controller Output Upper Limit"=→"Controller Output Upper Limit Readback":fxp<+/-,20,5>, "Kxx Output, Kxx*ex (V)"=→"Kxx Output, Kxx*ex (V)":fxp<+/-,58,25>, "Kyy Output, Kyy*ey (V)"=→"Kyy Output, Kyy*ey (V)":fxp<+/-,58,25>, "Kzz Output, Kzz*ez (V)"=→"Kzz Output, Kzz*ez (V)":fxp<+/-,58,25>)  [unwired: 1 out]
        n393 = xnode "Read/Write Control"("FPGA VI Reference In"=w1010, "error in"=w1011) -> ("error out"=w1008:errorcluster, "Controller loop iterations"=→"Controller loop iterations":i32, "Z Reference Loop iterations"=→"Z Reference Loop iterations":i32, "XY Reference Loop iterations"=→"XY Reference Loop iterations":i32, "FIFO loop iterations"=→"FIFO loop iterations":i32, "Trigger Generation Loop iterations"=→"Trigger Generation Loop iterations":i32, "Module output loop iterations"=→"Module output loop iterations":i32, "Plant output loop iterations"=→"Plant output loop iterations":i32, "Counter Loop iterations"=→"Counter Loop iterations":i32, "Outer Loop iterations"=→"Outer Loop iterations":i32)  [unwired: 1 out]
        n394 = xnode ("Read/Write Control")("FPGA VI Reference In"=w1010, "error in"=w1011) -> ("error out"=w1009:errorcluster, "Mod4/DIO0"=→"Mod4/DIO0":bool, "Mod4/DIO1"=→"Mod4/DIO1":bool, "Mod4/DIO2"=→"Mod4/DIO2":bool, "Mod4/DIO3"=→"Mod4/DIO3":bool, "Mod5/DIO0"=→"Mod5/DIO0":bool, "Mod5/DIO1"=→"Mod5/DIO1":bool, "Mod5/DIO2"=→"Mod5/DIO2":bool, "Mod5/DIO3"=→"Mod5/DIO3":bool, "Mod6/DIO0"=→"Mod6/DIO0":bool, "Mod6/DIO1"=→"Mod6/DIO1":bool, "Mod6/DIO2"=→"Mod6/DIO2":bool, "Mod6/DIO3"=→"Mod6/DIO3":bool, "Optics X Stage Displacement raw (nm)"=w995:fxp<+/-,32,16>, "Optics Y Stage Displacement raw (nm)"=w994:fxp<+/-,32,16>, "Optics Z Stage Displacement raw (nm)"=w993:fxp<+/-,32,16>, "Measured Datalog Period (Ticks)"=w999:u32, "Measured Counter Time Period (Ticks)"=w1000:u32)  [unwired: 1 out]
        "Measured Datalog Time Period (Ticks)" <- w999
        "Measured Counter Time Period (Ticks)" <- w1000
        "Optics X Stage Displacement (nm)" <- w995
        "Optics Y Stage Displacement (nm)" <- w994
        "Optics Z Stage Displacement (nm)" <- w993
        n395 = xnode "Read/Write Control"("FPGA VI Reference In"=w1010, "error in"=w1011) -> ("error out"=w1023:errorcluster, "X-Stage Input In Range?"=→"X-Stage Input In Range?":bool, "Y-Stage Input In Range?"=→"Y-Stage Input In Range?":bool, "Z-Stage Input In Range?"=→"Z-Stage Input In Range?":bool, "Measured Controller Loop Period (Ticks)"=w1063:u32, "Measured Module Output Loop Period (Ticks)"=w1062:u32, "Measured Plant Output Loop Period (Ticks)"=w1061:u32)  [unwired: 1 out]
        "Measured Controller Time Period (Ticks)" <- w1063
        "Measured Controller Output Time Period (Ticks)" <- w1062
        "Measured Plant Output Time Period (Ticks)" <- w1061
        n396 = xnode "Read/Write Control"("FPGA VI Reference In"=w1010, "error in"=w1011) -> ("error out"=w1024:errorcluster, "Measured XY Reference Loop Period (ticks)"=w1050:u32, "Measured Z Reference Loop Period (ticks)"=w1047:u32, "Measured Trigger Generation Loop Period (Ticks)"=w989:u32)  [unwired: 1 out]
        "Measured XY Reference Time Period (Ticks)" <- w1050
        "Measured Z Reference Time Period (Ticks)" <- w1047
        "Measured Trigger Gen Time Period (Ticks)" <- w989
        n397 = shared-variable "RT CompactRIO Target\\RT_EPICS_Shared_Variables.lvlib\\2iddVELO:VP:FPGA_State"(w1018) -> ()  [unwired: 1 in, 1 out]
        n398 = call "Convert Measured Rate.vi"("FPGA Clock Rate (Hz)"=w1043, "Measured Reference Time Period (Ticks)"=w1000) -> ("Measured Reference Loop Rate (kHz)"=w1041:dbl, "Measured Reference Loop Period (us)"=→"Measured Counter Loop Rate (us)":dbl)
        n399 = call "Convert Measured Rate.vi"("FPGA Clock Rate (Hz)"=w1043, "Measured Reference Time Period (Ticks)"=w999) -> ("Measured Reference Loop Rate (kHz)"=→"Measured Datalog Loop Rate (kHz)":dbl, "Measured Reference Loop Period (us)"=→"Measured Datalog Loop Rate (us)":dbl)
        n400 = call "Convert Measured Rate.vi"("FPGA Clock Rate (Hz)"=w1060, "Measured Reference Time Period (Ticks)"=w1063) -> ("Measured Reference Loop Rate (kHz)"=→"Measured Controller Loop Rate (kHz)":dbl, "Measured Reference Loop Period (us)"=→"Measured Controller Loop Rate (us)":dbl)
        n401 = call "Convert Measured Rate.vi"("FPGA Clock Rate (Hz)"=w1060, "Measured Reference Time Period (Ticks)"=w1061) -> ("Measured Reference Loop Rate (kHz)"=→"Measured Plant Output Loop Rate (kHz)":dbl, "Measured Reference Loop Period (us)"=→"Measured Plant Output Loop Rate (us)":dbl)
        n402 = call "Convert Measured Rate.vi"("FPGA Clock Rate (Hz)"=w1060, "Measured Reference Time Period (Ticks)"=w1062) -> ("Measured Reference Loop Rate (kHz)"=→"Measured Controller Output Loop Rate (kHz)":dbl, "Measured Reference Loop Period (us)"=→"Measured Controller Output Loop Rate (us)":dbl)
        n403 = call "Convert Measured Rate.vi"("FPGA Clock Rate (Hz)"=w990, "Measured Reference Time Period (Ticks)"=w989) -> ("Measured Reference Loop Rate (kHz)"=→"Measured Trigger Gen Loop Rate (kHz)":dbl, "Measured Reference Loop Period (us)"=→"Measured Trigger Gen Loop Rate (us)":dbl)
        n404 = call "Convert Measured Rate.vi"("FPGA Clock Rate (Hz)"=w990, "Measured Reference Time Period (Ticks)"=w1047) -> ("Measured Reference Loop Rate (kHz)"=→"Measured Z Reference Loop Rate (kHz)":dbl, "Measured Reference Loop Period (us)"=→"Measured Z Reference Loop Rate (us)":dbl)
        n405 = call "Convert Measured Rate.vi"("FPGA Clock Rate (Hz)"=w990, "Measured Reference Time Period (Ticks)"=w1050) -> ("Measured Reference Loop Rate (kHz)"=→"Measured XY Reference Loop Rate (kHz)":dbl, "Measured Reference Loop Period (us)"=→"Measured XY Reference Loop Rate (us)":dbl)
        n406 = Divide(x=w1041, y=1000.0) -> (x/y=→"Measured Counter Loop Rate (MHz)":dbl)
        n407 = To Double Precision Float(number=w993) -> (double precision float=w996:dbl)
        n408 = To Double Precision Float(number=w995) -> (double precision float=w998:dbl)
        n409 = To Double Precision Float(number=w994) -> (double precision float=w997:dbl)
        n410 = shared-variable "RT CompactRIO Target\\RT_EPICS_Shared_Variables.lvlib\\2iddVELO:LabView:ZPY_Readback"(w997) -> ()  [unwired: 1 in, 1 out]
        n411 = shared-variable "RT CompactRIO Target\\RT_EPICS_Shared_Variables.lvlib\\2iddVELO:LabView:ZPX_Readback"(w998) -> ()  [unwired: 1 in, 1 out]
        n412 = shared-variable "RT CompactRIO Target\\RT_EPICS_Shared_Variables.lvlib\\2iddVELO:LabView:ZPZ_Readback"(w996) -> ()  [unwired: 1 in, 1 out]
        n413 = Merge Errors(w1023, w1024, w1015, w1008, w1009) -> (w1022:errorcluster)
        "Readback error" <- w1022
        n414 = shared-variable ".\\Interloop communication.lvlib\\Readback Loop Error"(w1022) -> ()  [unwired: 1 in, 1 out]
      }
    }
    n415 = shared-variable ".\\Interloop communication.lvlib\\Stop System"() -> (w970:bool)  [unwired: 1 in, 1 out]
    n416 = Wait (ms)(milliseconds to wait=w971) -> ()  [unwired: 1 out]
    "Readback loop Iterations" <- w972
  }
  n417 = while {
    tunnel: w5 -> [w1073]
    shift-right: [w1072] -> _
    shift-left: Stream_SM_states."Open endpoint" ("f") -> [w1074]
    tunnel: [w1067] -> w6
    shift-right: [w1065] -> _
    shift-left: 0 -> [w1066]
    i -> [w1070]
    stop <- w1071 stop-if-true
    # "Error stream writer loop"
    n418 = global read "Error stream writer.vi" "Error stream writer"() -> (w1069:refnum<k21>)
    n419 = case shown="\"Open endpoint\", Default" w1074 {
      tunnel: w1069 -> [_ w1103 w1132 _]
      tunnel: w1073 -> [_ w1097 _ w1147]
      tunnel: [w1080 w1100 Stream_SM_states."Open endpoint" ("f") w1145] -> w1072
      tunnel: [_ _ _ w1136] -> w1071
      tunnel: [w1079 w1099 w1128 w1135] -> w1068
      tunnel: w1066 -> [w1075 w1096 w1127 w1134]
      tunnel: [w1075 w1095 w1127 w1134] -> w1065
      frame "Open endpoint", Default {
        w1078 = errorcluster {"status"=FALSE, "code"=0, "source"=""} ("error in (no error)")
        n420 = Create Network Stream Writer Endpoint(5:1000 ("timeout in ms (-1)"), 7:100000 ("writer buffer size"), 8:w1078, 9:w1078, 11:"/error/writer" ("reader url")) -> (0:w1081:errorcluster, 3:w1077:refnum<k21>)  [unwired: 2 in]
        n421 = case shown="No Error" w1081 {
          selector: w1081 -> [w1086 w1089]
          tunnel: [Stream_SM_states."Wait" Stream_SM_states."Open endpoint"] -> w1080
          tunnel: [w1086 w1088] -> w1079
          tunnel: w1077 -> [w1085 w1091]
          tunnel: [w1085 refnum<k21> refnum ("reader url")] -> w1076
          frame No Error {
          }
          frame Error {
            n422 = Flush Stream(8:w1089, 11:w1091) -> (0:w1092:errorcluster, 3:w1090:refnum<k21>)  [unwired: 2 in, 1 out]
            n423 = Destroy Stream Endpoint(8:w1092, 11:w1090) -> (0:w1088:errorcluster)
          }
        }
        n424 = global write "Error stream writer.vi" "Error stream writer"(w1076) -> ()
      }
      frame "ReadWrite" {
        n425 = property class="Network Stream Endpoint"(reference=w1103) -> (reference out=w1102:refnum<k21>, error out=w1101:errorcluster, "Connected"=w1098:bool)  [unwired: 1 in]
        "Error stream writer connection" <- w1098
        n426 = case shown="Error" w1101 {
          selector: w1101 -> [_ w1126]
          tunnel: [w1107 w1126] -> w1099
          tunnel: w1102 -> [w1111 _]
          tunnel: w1098 -> [w1110 _]
          tunnel: [w1108 Stream_SM_states."Destroy endpoint"] -> w1100
          tunnel: w1097 -> [w1106 _]
          tunnel: w1096 -> [w1105 w1124]
          tunnel: [w1104 w1124] -> w1095
          frame No Error {
            n427 = case shown="True" w1110 {
              tunnel: [errorcluster {"status"=FALSE, "code"=0, "source"=""} ("error IO") w1123] -> w1109
              tunnel: w1111 -> [_ w1122]
              tunnel: w1106 -> [_ w1121]
              tunnel: w1105 -> [w1116 w1119]
              tunnel: [w1116 w1118] -> w1104
              frame False {
              }
              frame True {
                n428 = Increment(x=w1119) -> (x+1=w1118:i32)
                n429 = Dequeue Element(queue=w1121) -> (element=w1120:errorcluster)  [unwired: 2 in, 3 out]
                n430 = shared-variable-write(w1122, w1120) -> (w1123:errorcluster)  [unwired: 2 in, 2 out]
              }
            }
            n431 = case shown="No Error" w1109 {
              selector: w1109 -> [w1112 w1114]
              tunnel: [Stream_SM_states."Wait" Stream_SM_states."Destroy endpoint"] -> w1108
              tunnel: [w1112 w1114] -> w1107
              frame No Error {
              }
              frame Error {
              }
            }
          }
          frame Error {
          }
        }
      }
      frame "Destroy endpoint" {
        n432 = Flush Stream(11:w1132) -> (0:w1130:errorcluster, 3:w1131:refnum<k21>)  [unwired: 3 in, 1 out]
        n433 = Destroy Stream Endpoint(8:w1130, 11:w1131) -> (0:w1128:errorcluster)
      }
      frame "Wait" {
        n434 = Get Queue Status(queue=w1147) -> (error out=w1135:errorcluster, # elements in queue=w1133:i32)  [unwired: 2 in, 6 out]
        n435 = Greater Than 0?(x=w1133) -> (x > 0?=w1146:bool)
        n436 = shared-variable ".\\Interloop communication.lvlib\\Stop System"() -> (w1138:bool)  [unwired: 1 in, 1 out]
        n437 = Select(t=Stream_SM_states."ReadWrite", s=w1146, f=Stream_SM_states."Wait") -> (s? t:f=w1145:T13)
        n438 = local read "Fly scan loop dt"() -> (w1141:i64)
        n439 = Equal To 0?(x=w1133) -> (x = 0?=w1137:bool)
        n440 = And(x=w1138, y=w1137) -> (x .and. y?=w1136:bool)
        n441 = Divide(x=w1141, y=i64 2) -> (x/y=w1140:dbl)
        n442 = To Unsigned Long Integer(number=w1140) -> (unsigned 32bit integer=w1142:u32)
        n443 = Wait Until Next ms Multiple(millisecond multiple=w1142) -> ()  [unwired: 1 out]
      }
    }
    "Error stream sends" <- w1065
    n444 = shared-variable ".\\Interloop communication.lvlib\\Error stream writer error"(w1068) -> ()  [unwired: 1 in, 1 out]
    n445 = call <vilib>:"Clear Errors.vi"("error in (no error)"=w1068) -> ("error out"=w1067:errorcluster)  [unwired: 5 in, 1 out]
    "Error stream writer iterations" <- w1070
    "Error stream state" <- w1074
  }
  n446 = Release Queue(queue=w5, error in (no error)=w6) -> ()  [unwired: 1 in, 3 out]
  n447 = Release Queue(queue=w3, error in (no error)=w4) -> ()  [unwired: 1 in, 3 out]
  n448 = node-c288(w20) -> (→"Timed Loop (end error)":errorcluster, →"Iteration Duration RT Timed-Loop":i64)
  n449 = Release Queue(queue=w11, error in (no error)=w15) -> ()  [unwired: 1 in, 3 out]
